vi "parking_ung2.vi"() -> ()   [LabVIEW 2012]
uses:
  G_SEN.vi
  G_NAV.vi
  G_PATH.vi
  G_VEH.vi
panel:
  out "M6006":T1={"GPSTime"=22892800.0, "attitude[2]"=-0.6123908, "lcc[0]"=-970.47205, "lcc[1]"=200.52362, "heading_GPS"=-0.6106907} {"GPSTime" format="%#_6f"}
  out "parkingpoint":dbl[][](array[numeric])=[[457.5136078182356, -783.1010211912842, 0.7436341447060439], [464.87374009628, -776.3313496446219, 0.7436341447060439], [466.7137731657911, -774.6389317579564, 0.7436341447060439], [468.5538062353022, -772.9465138712908, 0.3219638657386641], [475.6187081476555, -773.2417442369818, -0.09970641322871643], [485.5690424693232, -774.2371571598643, -0.09970641322871643]]
  out "max cost":i32=34
  out "sensor_obs":dbl[][](array[numeric])
  out "sensor_lane":dbl[][](array[numeric])=[[-17.75, -3.75, 0.0], [-17.5, -4.25, 0.0], [-17.5, -4.0, 0.0], [-17.25, -4.25, 0.0], [-14.5, -3.25, 0.0], [-14.25, -4.0, 0.0], [-14.25, -3.75, 0.0], [-14.25, -3.5, 0.0], [-13.0, -13.5, 0.0], [-12.0, -3.25, 0.0], [-11.75, -3.5, 0.0], [-11.25, 4.75, 0.0], [-11.25, 5.0, 0.0], [-10.0, -3.25, 0.0], [-9.75, -6.0, 0.0], [-9.75, -5.75, 0.0], [-9.75, -5.5, 0.0], [-9.75, 4.25, 0.0], [-9.5, -4.5, 0.0], [-9.25, -12.25, 0.0], [-9.25, -9.5, 0.0], [-9.25, -9.25, 0.0], [-9.25, -9.0, 0.0], [-9.25, -4.75, 0.0], [-9.25, -4.5, 0.0], [-9.0, -12.25, 0.0], [-9.0, -7.5, 0.0], [-9.0, -4.0, 0.0], [-8.75, -12.5, 0.0], [-8.75, -11.0, 0.0], [-8.75, 2.75, 0.0], [-8.5, -12.5, 0.0], [-8.5, -7.25, 0.0], [-8.5, -5.75, 0.0], [-8.5, -5.5, 0.0], [-8.5, -3.25, 0.0], [-8.25, 4.5, 0.0], [-7.75, 2.75, 0.0], [-7.75, 3.0, 0.0], [-7.5, -8.75, 0.0], [-7.25, -11.75, 0.0], [-7.25, -8.75, 0.0], [-7.25, 4.5, 0.0], [-7.0, -12.0, 0.0], [-7.0, -11.75, 0.0], [-7.0, -7.0, 0.0], [-7.0, -5.25, 0.0], [-6.75, -7.0, 0.0], [-6.75, -5.5, 0.0], [-6.75, 3.25, 0.0], [-6.75, 3.5, 0.0], [-6.75, 3.75, 0.0], [-6.75, 7.25, 0.0], [-6.75, 9.25, 0.0], [-6.5, -7.25, 0.0], [-6.5, 7.5, 0.0], [-6.5, 7.75, 0.0], [-6.25, -7.5, 0.0], [-6.25, -7.25, 0.0], [-6.25, 4.75, 0.0], [-6.25, 5.0, 0.0], [-6.25, 6.25, 0.0], [-6.0, -11.75, 0.0], [-6.0, -9.75, 0.0], [-6.0, -9.5, 0.0], [-6.0, 5.0, 0.0], [-5.75, -11.75, 0.0], [-5.75, -9.75, 0.0], [-5.75, -5.25, 0.0], [-5.75, -5.0, 0.0], [-5.5, -11.75, 0.0], [-5.5, -5.25, 0.0], [-5.25, -11.75, 0.0], [-5.0, -11.75, 0.0], [-5.0, -8.25, 0.0], [-5.0, -3.75, 0.0], [-4.75, -11.75, 0.0], [-4.75, -8.5, 0.0], [-4.75, -8.25, 0.0], [-4.75, -6.0, 0.0], [-4.75, -5.0, 0.0], [-4.75, -4.75, 0.0], [-4.75, -4.0, 0.0], [-4.75, -3.75, 0.0], [-4.5, -11.75, 0.0], [-4.5, -7.25, 0.0], [-4.5, -6.0, 0.0], [-4.25, -11.5, 0.0], [-4.25, -8.75, 0.0], [-4.25, -8.5, 0.0], [-4.25, -7.25, 0.0], [-4.0, -10.5, 0.0], [-4.0, -8.75, 0.0], [-3.75, -10.5, 0.0], [-2.75, -11.0, 0.0], [-2.5, -11.0, 0.0], [-2.25, -11.0, 0.0], [-2.0, -18.0, 0.0], [-2.0, -11.0, 0.0], [-1.75, -11.0, 0.0], [-1.5, -18.0, 0.0], [-1.5, -11.0, 0.0], [-1.25, -18.0, 0.0], [-1.25, -11.0, 0.0], [-1.0, -18.0, 0.0], [-1.0, -12.25, 0.0], [-1.0, -11.0, 0.0], [-0.75, -18.0, 0.0], [-0.75, -12.5, 0.0], [-0.5, -18.0, 0.0], [-0.5, -12.5, 0.0], [1.75, -12.5, 0.0], [2.0, -12.5, 0.0], [2.0, 9.0, 0.0], [2.25, 6.5, 0.0], [2.25, 7.25, 0.0], [2.5, -17.5, 0.0], [2.5, -12.25, 0.0], [2.5, 4.5, 0.0], [2.5, 5.0, 0.0], [2.5, 5.25, 0.0], [2.5, 5.5, 0.0], [2.5, 6.0, 0.0], [2.5, 6.5, 0.0], [2.5, 7.25, 0.0], [2.75, -17.5, 0.0], [2.75, -12.25, 0.0], [2.75, -10.5, 0.0], [2.75, 2.75, 0.0], [2.75, 3.0, 0.0], [2.75, 3.25, 0.0], [2.75, 3.5, 0.0], [2.75, 3.75, 0.0], [2.75, 4.0, 0.0], [2.75, 4.5, 0.0], [2.75, 4.75, 0.0], [2.75, 5.0, 0.0], [2.75, 5.25, 0.0], [2.75, 7.0, 0.0], [3.0, -12.25, 0.0], [3.0, -12.0, 0.0], [3.0, -10.5, 0.0], [3.0, 2.75, 0.0], [3.0, 3.0, 0.0], [3.0, 3.25, 0.0], [3.0, 3.5, 0.0], [3.0, 4.5, 0.0], [3.0, 4.75, 0.0], [3.25, -17.5, 0.0], [3.25, -10.5, 0.0], [3.5, -10.5, 0.0], [3.5, 4.75, 0.0], [3.75, -17.5, 0.0], [3.75, -4.75, 0.0], [3.75, -4.0, 0.0], [3.75, -3.5, 0.0], [3.75, 7.25, 0.0], [4.0, -6.25, 0.0], [4.0, -5.25, 0.0], [4.0, -4.75, 0.0], [4.0, -4.5, 0.0], [4.0, -4.0, 0.0], [4.0, 4.75, 0.0], [4.0, 5.0, 0.0], [4.0, 7.25, 0.0], [4.25, -10.25, 0.0], [4.25, -8.5, 0.0], [4.25, -5.25, 0.0], [4.5, -10.25, 0.0], [4.5, -8.5, 0.0], [4.5, 5.0, 0.0], [4.75, -17.5, 0.0], [4.75, -10.25, 0.0], [4.75, 4.75, 0.0], [4.75, 5.0, 0.0], [5.0, -17.5, 0.0], [5.0, -10.0, 0.0], [5.25, -10.0, 0.0], [5.25, 5.0, 0.0], [5.5, -10.0, 0.0], [5.5, 5.0, 0.0], [5.75, -5.0, 0.0], [6.0, -5.0, 0.0], [6.0, 5.25, 0.0], [6.25, 5.0, 0.0], [6.25, 5.25, 0.0], [6.75, -17.25, 0.0], [6.75, -17.0, 0.0], [6.75, 4.75, 0.0], [7.0, 2.75, 0.0], [7.0, 5.25, 0.0], [7.0, 5.5, 0.0], [7.25, 4.5, 0.0], [7.25, 7.75, 0.0], [7.25, 8.75, 0.0], [7.25, 9.0, 0.0], [7.5, -4.75, 0.0], [7.5, 6.0, 0.0], [7.5, 7.75, 0.0], [7.75, -4.75, 0.0], [15.0, -19.25, 0.0], [15.25, -19.25, 0.0], [15.5, -19.0, 0.0], [16.0, -19.0, 0.0], [16.0, -10.25, 0.0], [16.5, -10.25, 0.0], [16.75, -10.0, 0.0], [17.25, -10.0, 0.0], [17.5, -8.75, 0.0], [17.75, -9.75, 0.0], [17.75, -9.5, 0.0], [18.0, -9.5, 0.0], [18.0, -9.25, 0.0], [18.25, -9.25, 0.0], [18.5, -9.0, 0.0], [18.75, -9.0, 0.0], [18.75, -8.75, 0.0], [19.0, -8.75, 0.0], [19.0, -8.5, 0.0], [19.25, -8.25, 0.0], [19.5, -8.25, 0.0]]
  out "box":dbl[][](array[numeric])=[[2.75, 2.75], [7.75, 2.7499999999999996], [7.75, 5.0], [2.7500000000000004, 5.0], [2.75, 2.75]]
  out "time":u32=1
  out "tic":u32=336066801
  out "XY Graph":cluster{"Y":dbl[], "Y":dbl[]}[](graph)=[{"Y"=[2.25, 2.25, 2.5, 2.5, 2.5, 2.75, 2.75, 3.0, 3.25, 3.25, 3.5, 3.5, 4.0, 4.0, 4.5, 4.5, 4.75, 4.75, 4.75, 5.0, 5.25], "Y"=[4.25, 4.5, 4.0, 4.25, 4.5, 3.75, 4.0, 3.75, 3.5, 3.75, 3.25, 3.5, 3.0, 3.25, 2.75, 3.0, 3.25, 3.5, 4.0, 4.0, 4.5]}, {"Y"=[-25.0, -25.0, -15.0, -13.75, -10.5, -9.75, -8.5, -8.25, -8.0, -7.5, -7.25, -7.0, -7.0, -6.75, -6.5, -6.25, -6.25, -6.0, -6.0, -6.0, -5.75, -5.0, -4.75, -4.75, -4.5, -4.25, -4.25, -4.25, -4.25, -4.0, -4.0, -4.0, -4.0, -4.0, -3.75, -3.75, -3.75, -3.75, -3.5, -3.5, -3.5, -3.25, -3.25, -3.25, -3.25, -3.25, -3.0, -3.0, -3.0, -3.0, -3.0, -2.75, -2.5, -2.5, -2.5, -2.25, -2.25, -2.25, -2.0, -2.0, -2.0, -2.0, -2.0, -1.75, -1.75, -1.75, -1.75, -1.5, -1.5, -1.5, -1.5, -1.25, -1.25, -1.0, -1.0, -1.0, -0.75, -0.75, -0.75, -0.5, -0.5, -0.5, -0.25, -0.25, 0.0, 0.25, 0.25, 0.5, 0.75, 1.0, 1.0, 1.25, 1.25, 1.5, 1.5, 1.5, 1.5, 1.5, 1.5, 1.5, 1.75, 1.75, 1.75, 1.75, 1.75, 1.75, 1.75, 2.0, 2.0, 2.0, 2.0, 2.0, 2.25, 2.25, 2.25, 2.25, 2.25, 2.25, 2.25, 2.5, 2.5, 2.5, 2.5, 2.5, 2.5, 2.75, 2.75, 2.75, 2.75, 3.0, 3.0, 3.25, 3.25, 3.25, 3.25, 3.25, 3.25, 3.5, 3.5, 3.5, 3.75, 4.0, 4.0, 4.0, 4.0, 4.25, 4.25, 4.5, 4.5, 4.75, 4.75, 4.75, 5.0, 5.25, 5.25, 5.5, 5.5, 5.5, 5.5, 5.75, 5.75, 6.0, 6.0, 6.0, 6.0, 6.0, 6.25, 6.25, 6.25, 6.5, 6.5, 6.5, 6.5, 6.5, 6.5, 6.5, 6.75, 6.75, 6.75, 6.75, 6.75, 7.0, 7.0, 7.0, 7.25, 7.25, 7.25, 7.25, 7.5, 7.5, 7.5, 7.5, 7.75, 7.75, 7.75, 7.75, 8.0, 8.0, 8.0, 8.0, 8.0, 8.25, 8.25, 8.25, 8.5, 8.5, 8.5, 8.5, 8.75, 8.75, 8.75, 9.0, 9.0, 9.0, 9.0, 9.0, 9.25, 9.25, 9.25, 9.25, 9.25, 9.25, 9.5, 9.5, 9.5, 9.5, 9.5, 9.5, 9.5, 9.75, 9.75, 9.75, 9.75, 9.75, 10.0, 10.0, 10.0, 10.0, 10.0, 10.0, 10.25, 10.25, 10.25, 10.25, 10.25, 10.25, 10.5, 10.5, 10.5, 10.5, 10.75, 10.75, 10.75, 11.0, 11.0, 11.0, 11.0, 11.0, 11.25, 11.25, 11.25, 11.5, 11.75, 12.0, 14.25, 14.5, 14.75, 14.75, 14.75, 14.75, 14.75, 15.0, 15.0, 15.25, 15.25, 15.25, 15.25, 15.5, 15.5, 15.5, 15.5, 15.75, 15.75, 15.75, 16.0, 16.0, 16.25, 16.25, 16.5, 16.5, 17.0, 17.25, 17.5, 17.5, 17.75, 17.75, 17.75, 17.75, 18.0, 18.0, 18.0, 18.0, 18.0, 18.0, 18.0, 18.0, 18.25, 18.25, 18.25, 18.25, 18.5, 18.5, 18.5, 18.75, 18.75, 18.75, 19.0, 19.0, 19.0, 19.0, 19.0, 19.25, 19.25, 19.25, 19.25, 19.25, 19.25, 19.25, 19.5, 19.5, 19.5, 19.5, 19.5, 19.5, 19.5, 19.75, 19.75, 19.75, 19.75, 19.75, 19.75, 20.0, 20.0, 20.0, 20.0, 20.0, 20.0, 20.25, 20.25, 20.25, 20.25, 20.25, 20.5, 20.5, 20.5, 20.75, 20.75, 21.0, 21.0, 21.0, 21.5, 21.5, 21.5, 21.5, 22.0, 22.25, 22.5, 22.5, 22.5, 22.5, 22.75, 22.75, 23.0, 23.25, 23.5, 23.75, 24.0, 24.0, 24.0, 24.0, 24.25, 24.25, 24.5, 24.5, 24.75, 24.75, 24.75, -1.75, -1.25, -1.0, -0.5, 0.0, -3.0, -3.0, -1.75, 0.25], "Y"=[6.5, 22.75, -12.0, -8.5, -4.25, -13.75, -11.0, -11.25, -11.25, 9.5, -9.25, -9.5, -9.25, -9.5, -7.75, -8.0, 8.75, -8.0, -6.75, 8.75, -6.75, 8.0, -6.25, 8.0, -5.25, -5.5, -5.25, 13.5, 13.75, -4.75, 7.5, 8.5, 8.75, 13.5, -4.25, 7.5, 8.75, 13.25, -3.75, 13.0, 13.25, -7.5, -3.5, -3.25, 7.0, 13.0, -8.5, -8.0, -7.5, 7.0, 7.25, -8.0, -7.75, -7.0, 6.75, -6.25, -3.25, 6.75, -6.25, -5.5, -3.25, 6.75, 7.0, -5.5, -5.0, -3.5, 6.25, -5.0, -4.75, -3.5, 7.75, -4.75, -4.25, -9.25, -7.25, -4.25, -7.25, -6.25, 5.75, -9.25, -7.25, -6.25, -9.25, 5.5, 5.5, 5.25, 5.5, 5.0, -5.0, -7.0, -5.0, -10.75, -6.25, -13.5, -13.25, -11.25, -10.25, -6.25, -6.0, -5.5, -13.0, -11.5, -11.25, -10.75, -9.0, -7.75, -5.5, -12.75, -11.5, -10.75, -9.0, -7.75, -11.5, -11.25, -10.5, -6.0, -5.75, 4.25, 4.5, -11.25, -10.5, -5.75, 4.0, 4.25, 4.5, -11.0, -10.25, 3.75, 4.0, -6.5, 3.75, -9.5, -6.5, -6.25, 3.5, 3.75, 6.0, -9.0, 3.25, 3.5, 7.0, -7.0, 3.0, 3.25, 7.75, -7.0, 7.75, 2.75, 3.0, 3.25, 3.5, 4.0, 4.0, -5.0, 4.5, -5.0, -4.75, 5.0, 5.25, -4.75, -4.5, -5.0, -4.5, -4.25, 6.0, 6.75, -5.0, -4.25, -4.0, -19.25, -19.0, -4.0, -3.75, -3.5, 6.75, 7.0, -19.0, -18.75, -3.5, -3.25, 7.5, -19.0, -5.25, 7.25, -19.0, -18.75, -5.25, -5.0, -18.75, -18.25, -5.0, -4.75, -18.25, -18.0, -4.75, -4.5, -18.0, -17.75, -5.75, -4.25, -4.0, -5.5, -4.0, -3.75, -5.25, -5.0, -3.5, -3.25, -17.25, -6.75, -4.75, -13.25, -6.75, -6.5, -4.75, -4.5, -13.0, -12.75, -6.5, -6.25, -4.25, -4.0, -12.75, -12.5, -8.75, -6.0, -4.0, -3.75, -3.5, -12.5, -12.25, -5.75, -5.5, -3.25, -12.25, -12.0, -5.5, -5.25, 2.75, 3.0, -12.0, -11.75, -11.5, -5.25, -5.0, -4.75, -11.5, -11.25, -4.75, -4.5, -11.0, -4.5, -4.25, -10.75, -10.5, -10.25, -3.75, -3.5, -10.25, -10.0, -3.25, -10.0, -6.0, -6.0, -13.25, -13.0, -13.0, -12.75, -12.5, -5.75, -5.5, -12.5, -5.5, -12.25, -12.0, -4.75, -4.5, -12.0, -11.75, -4.5, -4.25, -11.25, -4.25, -4.0, -10.75, -3.75, -10.5, -10.25, -10.25, -10.0, -9.5, 16.75, -8.75, 16.75, -8.75, 16.25, 16.5, 16.75, -8.5, -8.25, -8.0, 15.25, 15.5, 15.75, 16.0, 16.25, -8.0, -7.75, 15.25, 15.5, 2.75, 15.0, 15.25, -7.5, 3.0, 15.0, -7.25, -7.0, 3.5, 3.75, 4.0, -19.25, -6.75, -6.5, -6.25, 4.0, 4.25, 4.5, -19.25, -19.0, -18.75, -18.25, -6.5, -6.25, 4.5, -18.5, -18.25, -18.0, -17.75, 4.75, 5.0, -17.75, -17.25, -5.0, 5.25, 5.5, 5.75, -16.75, -5.0, 5.75, 6.0, 6.25, -16.75, -4.75, 6.5, -16.5, -4.5, -16.0, -15.75, -4.25, -15.25, -15.0, -4.0, -3.75, -15.0, -14.75, -14.75, -14.5, -14.25, -14.0, -14.0, -13.75, -13.5, -13.5, -12.25, -12.0, -12.0, -11.75, -11.5, -11.25, -11.75, -11.25, -11.0, 5.0, -10.0, 22.75, 23.0, 6.5, 6.0, 6.0, 5.75, 5.75, 10.25, 10.5, 7.75, 5.75]}, {"Y"=[1.0, 1.0, 1.0, 1.0, 1.0, 1.0, 1.0, 1.0, 1.0, 1.0, 1.0, 1.0, 1.0, 1.0, 1.0, 1.25, 1.25, 1.25, 1.25, 1.25, 1.25, 1.25, 1.25, 1.25, 1.25, 1.25, 1.25, 1.25, 1.25, 1.25, 1.25, 1.5, 1.5, 1.5, 1.5, 1.5, 1.5, 1.5, 1.5, 1.5, 1.5, 1.5, 1.5, 1.75, 1.75, 1.75, 1.75, 1.75, 1.75, 1.75, 1.75, 2.0, 2.0, 2.0, 2.0, 2.0, 2.0, 2.0, 2.0, 2.25, 2.25, 2.25, 2.25, 2.25, 2.25, 2.25, 2.25, 2.5, 2.5, 2.5, 2.5, 2.5, 2.5, 2.5, 2.5, 2.5, 2.5, 2.75, 2.75, 2.75, 2.75, 2.75, 2.75, 2.75, 2.75, 2.75, 2.75, 3.0, 3.0, 3.0, 3.0, 3.0, 3.0, 3.25, 3.25, 3.25, 3.5, 3.5, 3.5, 3.5, 3.75], "Y"=[5.0, 5.25, 5.5, 5.75, 6.0, 6.5, 7.0, 7.5, 7.75, 8.0, 8.25, 8.5, 9.0, 9.25, 9.5, 4.75, 5.0, 5.25, 5.5, 5.75, 6.0, 6.25, 6.5, 6.75, 7.5, 7.75, 8.0, 8.25, 8.5, 8.75, 9.0, 4.75, 5.0, 5.25, 5.5, 5.75, 6.0, 6.25, 6.5, 6.75, 8.5, 8.75, 9.0, 4.75, 5.0, 5.25, 5.5, 5.75, 6.75, 7.5, 9.0, 4.75, 5.0, 5.25, 5.5, 5.75, 6.75, 7.0, 7.5, 4.75, 5.0, 5.25, 5.5, 5.75, 6.5, 6.75, 7.5, 4.75, 5.0, 5.25, 5.5, 5.75, 6.0, 6.5, 7.25, 7.5, 9.75, 4.75, 5.0, 5.25, 5.5, 5.75, 6.0, 6.25, 6.5, 7.0, 7.25, 5.5, 6.0, 6.5, 6.75, 7.0, 7.25, 6.5, 6.75, 7.0, 6.5, 7.25, 7.5, 7.75, 7.25]}, {"Y"=[-24.75, -24.75, -24.75, -24.75, -24.5, -24.5, -24.5, -24.5, -24.25, -24.25, -24.25, -24.25, -24.25, -24.0, -24.0, -24.0, -24.0, -24.0, -24.0, -24.0, -24.0, -24.0, -23.75, -23.75, -23.75, -23.75, -23.75, -23.75, -23.75, -23.5, -23.5, -23.5, -23.5, -23.5, -23.5, -23.5, -23.5, -23.5, -23.5, -23.5, -23.25, -23.25, -23.25, -23.25, -23.25, -23.25, -23.25, -23.25, -23.25, -23.25, -23.0, -23.0, -23.0, -23.0, -23.0, -23.0, -23.0, -23.0, -22.75, -22.75, -22.75, -22.75, -22.75, -22.75, -22.75, -22.75, -22.75, -22.75, -22.5, -22.5, -22.5, -22.5, -22.5, -22.5, -22.5, -22.5, -22.5, -22.5, -22.5, -22.5, -22.5, -22.5, -22.25, -22.25, -22.25, -22.25, -22.25, -22.25, -22.25, -22.25, -22.25, -22.25, -22.25, -22.25, -22.25, -22.25, -22.25, -22.25, -22.25, -22.0, -22.0, -22.0, -22.0, -22.0, -22.0, -22.0, -22.0, -22.0, -22.0, -22.0, -21.75, -21.75, -21.75, -21.75, -21.5, -21.5, -21.5, -21.25, -21.25, -21.25, -21.25, -21.25, -21.0, -21.0, -21.0, -21.0, -21.0, -20.75, -20.75, -20.75, -20.75, -20.75, -20.75, -20.75, -20.5, -20.5, -20.0, -20.0, -19.75, -19.5, -19.25, -19.25, -19.25, -19.25, -19.0, -19.0, -19.0, -19.0, -18.75, -18.75, -18.75, -18.75, -18.75, -18.75, -18.5, -18.5, -18.5, -18.5, -18.5, -18.5, -18.5, -18.5, -18.5, -18.5, -18.5, -18.25, -18.25, -18.25, -18.25, -18.25, -18.25, -18.25, -18.25, -18.25, -18.25, -18.25, -18.25, -18.25, -18.25, -18.25, -18.0, -18.0, -18.0, -18.0, -18.0, -18.0, -18.0, -18.0, -18.0, -18.0, -18.0, -18.0, -18.0, -18.0, -18.0, -17.75, -17.75, -17.75, -17.75, -17.75, -17.75, -17.75, -17.75, -17.75, -17.75, -17.5, -17.5, -17.5, -17.5, -17.5, -17.5, -17.5, -17.5, -17.5, -17.5, -17.5, -17.25, -17.25, -17.25, -17.25, -17.25, -17.25, -17.25, -17.25, -17.25, -17.0, -17.0, -17.0, -17.0, -16.75, -16.75, -16.5, -16.0, -16.0, -16.0, -16.0, -15.75, -15.75, -15.75, -15.75, -15.75, -15.75, -15.75, -15.75, -15.75, -15.5, -15.5, -15.5, -15.5, -15.5, -15.5, -15.5, -15.5, -15.5, -15.25, -15.25, -15.25, -15.25, -15.25, -15.25, -15.25, -15.25, -15.0, -15.0, -15.0, -15.0, -15.0, -15.0, -15.0, -15.0, -15.0, -15.0, -14.75, -14.75, -14.75, -14.75, -14.75, -14.75, -14.75, -14.75, -14.75, -14.5, -14.5, -14.5, -14.25, -14.25, -14.25, -14.25, -14.0, -14.0, -14.0, -14.0, -14.0, -13.75, -13.75, -13.75, -13.75, -13.75, -13.75, -13.75, -13.75, -13.75, -13.5, -13.5, -13.5, -13.5, -13.5, -13.5, -13.5, -13.25, -13.25, -13.25, -13.25, -13.25, -13.25, -13.25, -13.0, -13.0, -13.0, -13.0, -13.0, -12.75, -12.75, -12.75, -12.75, -12.5, -12.5, -12.5, -12.5, -12.5, -12.5, -12.5, -12.5, -12.5, -12.25, -12.25, -12.25, -12.25, -12.25, -12.25, -12.25, -12.25, -12.25, -12.25, -12.25, -12.25, -12.25, -12.25, -12.25, -12.25, -12.25, -12.0, -12.0, -12.0, -12.0, -12.0, -12.0, -12.0, -12.0, -12.0, -12.0, -12.0, -12.0, -11.75, -11.75, -11.75, -11.75, -11.75, -11.75, -11.75, -11.75, -11.75, -11.75, -11.75, -11.75, -11.75, -11.75, -11.75, -11.75, -11.75, -11.75, -11.5, -11.5, -11.5, -11.5, -11.5, -11.5, -11.5, -11.5, -11.5, -11.5, -11.5, -11.25, -11.25, -11.25, -11.25, -11.25, -11.25, -11.25, -11.25, -11.25, -11.0, -11.0, -11.0, -11.0, -11.0, -11.0, -11.0, -11.0, -11.0, -11.0, -11.0, -11.0, -10.75, -10.75, -10.75, -10.75, -10.75, -10.75, -10.75, -10.75, -10.75, -10.75, -10.75, -10.5, -10.5, -10.5, -10.5, -10.5, -10.5, -10.5, -10.25, -10.25, -10.25, -10.25, -10.25, -10.0, -10.0, -10.0, -10.0, -10.0, -9.75, -9.75, -9.75, -9.5, -9.5, -9.25, -9.25, -9.25, -9.0, -9.0, -9.0, -9.0, -8.75, -8.75, -8.75, -8.75, -8.5, -8.5, -8.5, -8.25, -8.25, -8.25, -8.25, -8.25, -8.25, -8.0, -8.0, -8.0, -8.0, -8.0, -8.0, -7.75, -7.75, -7.75, -7.75, -7.75, -7.5, -7.5, -7.5, -7.5, -7.5, -7.5, -7.25, -7.25, -7.25, -7.25, -7.25, -7.0, -7.0, -7.0, -7.0, -7.0, -7.0, -7.0, -7.0, -7.0, -6.75, -6.75, -6.75, -6.75, -6.75, -6.5, -6.5, -6.5, -6.5, -6.5, -6.25, -6.25, -6.25, -6.25, -6.25, -6.0, -6.0, -6.0, -6.0, -6.0, -6.0, -5.75, -5.75, -5.75, -5.75, -5.75, -5.75, -5.75, -5.75, -5.75, -5.75, -5.75, -5.5, -5.5, -5.5, -5.5, -5.5, -5.5, -5.5, -5.5, -5.5, -5.5, -5.5, -5.5, -5.5, -5.5, -5.25, -5.25, -5.25, -5.25, -5.25, -5.25, -5.25, -5.25, -5.25, -5.25, -5.25, -5.0, -5.0, -5.0, -5.0, -5.0, -5.0, -5.0, -5.0, -5.0, -5.0, -5.0, -4.75, -4.75, -4.75, -4.75, -4.75, -4.75, -4.75, -4.75, -4.75, -4.75, -4.75, -4.75, -4.75, -4.75, -4.75, -4.5, -4.5, -4.5, -4.5, -4.5, -4.5, -4.5, -4.5, -4.5, -4.25, -4.25, -4.25, -4.25, -4.25, -4.25, -4.25, -4.25, -4.0, -4.0, -4.0, -4.0, -4.0, -4.0, -4.0, -4.0, -4.0, -4.0, -4.0, -3.75, -3.75, -3.75, -3.75, -3.75, -3.75, -3.75, -3.75, -3.75, -3.75, -3.75, -3.5, -3.5, -3.5, -3.5, -3.5, -3.5, -3.5, -3.5, -3.5, -3.25, -3.25, -3.25, -3.25, -3.25, -3.25, -3.25, -3.25, -3.25, -3.25, -3.25, -3.25, -3.0, -3.0, -3.0, -3.0, -3.0, -3.0, -3.0, -3.0, -3.0, -3.0, -3.0, -2.75, -2.75, -2.75, -2.75, -2.75, -2.75, -2.75, -2.75, -2.75, -2.75, -2.75, -2.75, -2.75, -2.75, -2.75, -2.5, -2.5, -2.5, -2.5, -2.5, -2.5, -2.5, -2.5, -2.5, -2.5, -2.5, -2.5, -2.25, -2.25, -2.25, -2.25, -2.25, -2.25, -2.25, -2.25, -2.25, -2.25, -2.25, -2.25, -2.0, -2.0, -2.0, -2.0, -2.0, -2.0, -2.0, -2.0, -2.0, -2.0, -2.0, -2.0, -2.0, -2.0, -2.0, -1.75, -1.75, -1.75, -1.75, -1.75, -1.75, -1.75, -1.75, -1.75, -1.75, -1.75, -1.75, -1.5, -1.5, -1.5, -1.5, -1.5, -1.5, -1.5, -1.5, -1.5, -1.5, -1.5, -1.5, -1.5, -1.5, -1.5, -1.5, -1.5, -1.5, -1.25, -1.25, -1.25, -1.25, -1.25, -1.25, -1.25, -1.25, -1.25, -1.25, -1.25, -1.25, -1.25, -1.25, -1.25, -1.25, -1.0, -1.0, -1.0, -1.0, -1.0, -1.0, -1.0, -1.0, -1.0, -1.0, -1.0, -1.0, -1.0, -1.0, -0.75, -0.75, -0.75, -0.75, -0.75, -0.75, -0.75, -0.75, -0.75, -0.75, -0.75, -0.75, -0.75, -0.75, -0.5, -0.5, -0.5, -0.5, -0.5, -0.5, -0.5, -0.5, -0.5, -0.5, -0.5, -0.5, -0.5, -0.5, -0.25, -0.25, -0.25, -0.25, -0.25, -0.25, -0.25, -0.25, -0.25, -0.25, 0.0, 0.0, 0.0, 0.0, 0.0, 0.0, 0.0, 0.0, 0.0, 0.0, 0.0, 0.0, 0.25, 0.25, 0.25, 0.25, 0.25, 0.25, 0.25, 0.25, 0.25, 0.25, 0.25, 0.25, 0.25, 0.5, 0.5, 0.5, 0.5, 0.5, 0.5, 0.5, 0.5, 0.5, 0.5, 0.75, 0.75, 0.75, 0.75, 0.75, 0.75, 0.75, 0.75, 0.75, 0.75, 0.75, 0.75, 0.75, 1.0, 1.0, 1.0, 1.0, 1.0, 1.0, 1.0, 1.0, 1.0, 1.0, 1.0, 1.0, 1.0, 1.0, 1.0, 1.25, 1.25, 1.25, 1.25, 1.25, 1.25, 1.25, 1.25, 1.25, 1.25, 1.25, 1.25, 1.25, 1.25, 1.25, 1.25, 1.25, 1.25, 1.5, 1.5, 1.5, 1.5, 1.5, 1.5, 1.5, 1.5, 1.5, 1.5, 1.5, 1.5, 1.5, 1.5, 1.75, 1.75, 1.75, 1.75, 1.75, 1.75, 1.75, 1.75, 1.75, 1.75, 1.75, 1.75, 1.75, 2.0, 2.0, 2.0, 2.0, 2.0, 2.0, 2.0, 2.0, 2.0, 2.0, 2.0, 2.0, 2.0, 2.0, 2.0, 2.0, 2.0, 2.0, 2.25, 2.25, 2.25, 2.25, 2.25, 2.25, 2.25, 2.25, 2.25, 2.25, 2.25, 2.25, 2.25, 2.25, 2.25, 2.25, 2.25, 2.25, 2.5, 2.5, 2.5, 2.5, 2.5, 2.5, 2.5, 2.5, 2.5, 2.5, 2.5, 2.5, 2.5, 2.5, 2.5, 2.5, 2.5, 2.5, 2.5, 2.75, 2.75, 2.75, 2.75, 2.75, 2.75, 2.75, 2.75, 2.75, 2.75, 2.75, 2.75, 2.75, 2.75, 2.75, 2.75, 2.75, 2.75, 2.75, 2.75, 2.75, 3.0, 3.0, 3.0, 3.0, 3.0, 3.0, 3.0, 3.0, 3.0, 3.0, 3.0, 3.0, 3.0, 3.0, 3.0, 3.25, 3.25, 3.25, 3.25, 3.25, 3.25, 3.25, 3.25, 3.25, 3.25, 3.25, 3.25, 3.25, 3.5, 3.5, 3.5, 3.5, 3.5, 3.5, 3.5, 3.5, 3.5, 3.5, 3.5, 3.5, 3.5, 3.5, 3.5, 3.75, 3.75, 3.75, 3.75, 3.75, 3.75, 3.75, 3.75, 3.75, 3.75, 3.75, 4.0, 4.0, 4.0, 4.0, 4.0, 4.0, 4.0, 4.0, 4.0, 4.0, 4.25, 4.25, 4.25, 4.25, 4.25, 4.25, 4.25, 4.25, 4.25, 4.5, 4.5, 4.5, 4.5, 4.5, 4.5, 4.5, 4.5, 4.5, 4.5, 4.5, 4.75, 4.75, 4.75, 4.75, 4.75, 4.75, 4.75, 4.75, 4.75, 4.75, 5.0, 5.0, 5.0, 5.0, 5.0, 5.0, 5.0, 5.0, 5.0, 5.0, 5.0, 5.0, 5.25, 5.25, 5.25, 5.25, 5.25, 5.25, 5.25, 5.25, 5.25, 5.25, 5.25, 5.25, 5.25, 5.25, 5.25, 5.5, 5.5, 5.5, 5.5, 5.5, 5.5, 5.5, 5.5, 5.5, 5.5, 5.5, 5.5, 5.5, 5.5, 5.5, 5.5, 5.5, 5.5, 5.5, 5.5, 5.5, 5.5, 5.5, 5.75, 5.75, 5.75, 5.75, 5.75, 5.75, 5.75, 5.75, 5.75, 5.75, 5.75, 5.75, 5.75, 5.75, 5.75, 5.75, 5.75, 5.75, 5.75, 5.75, 5.75, 5.75, 5.75, 5.75, 5.75, 5.75, 6.0, 6.0, 6.0, 6.0, 6.0, 6.0, 6.0, 6.0, 6.0, 6.0, 6.0, 6.0, 6.0, 6.0, 6.0, 6.0, 6.0, 6.0, 6.0, 6.0, 6.0, 6.0, 6.0, 6.0, 6.0, 6.25, 6.25, 6.25, 6.25, 6.25, 6.25, 6.25, 6.25, 6.25, 6.25, 6.25, 6.25, 6.25, 6.25, 6.5, 6.5, 6.5, 6.5, 6.5, 6.5, 6.5, 6.5, 6.5, 6.5, 6.5, 6.5, 6.5, 6.5, 6.5, 6.5, 6.5, 6.5, 6.5, 6.5, 6.5, 6.5, 6.75, 6.75, 6.75, 6.75, 6.75, 6.75, 6.75, 6.75, 6.75, 6.75, 6.75, 6.75, 6.75, 6.75, 6.75, 6.75, 6.75, 7.0, 7.0, 7.0, 7.0, 7.0, 7.0, 7.0, 7.0, 7.0, 7.0, 7.0, 7.0, 7.0, 7.0, 7.0, 7.0, 7.0, 7.25, 7.25, 7.25, 7.25, 7.25, 7.25, 7.25, 7.25, 7.25, 7.25, 7.25, 7.25, 7.25, 7.25, 7.25, 7.5, 7.5, 7.5, 7.5, 7.5, 7.5, 7.5, 7.5, 7.5, 7.5, 7.5, 7.5, 7.5, 7.75, 7.75, 7.75, 7.75, 7.75, 7.75, 7.75, 7.75, 7.75, 7.75, 7.75, 7.75, 7.75, 7.75, 8.0, 8.0, 8.0, 8.0, 8.0, 8.0, 8.0, 8.0, 8.25, 8.25, 8.25, 8.25, 8.25, 8.25, 8.25, 8.5, 8.5, 8.5, 8.5, 8.5, 8.5, 8.5, 8.5, 8.5, 8.75, 8.75, 8.75, 8.75, 8.75, 8.75, 8.75, 8.75, 8.75, 8.75, 8.75, 8.75, 9.0, 9.0, 9.0, 9.0, 9.0, 9.0, 9.0, 9.0, 9.0, 9.0, 9.0, 9.0, 9.0, 9.0, 9.0, 9.25, 9.25, 9.25, 9.25, 9.25, 9.25, 9.25, 9.25, 9.25, 9.25, 9.25, 9.25, 9.25, 9.25, 9.25, 9.25, 9.25, 9.25, 9.25, 9.25, 9.25, 9.5, 9.5, 9.5, 9.5, 9.5, 9.5, 9.5, 9.5, 9.5, 9.5, 9.5, 9.5, 9.5, 9.5, 9.75, 9.75, 9.75, 9.75, 9.75, 10.0, 10.0, 10.0, 10.0, 10.0, 10.25, 10.25, 10.25, 10.25, 10.25, 10.25, 10.25, 10.25, 10.25, 10.25, 10.25, 10.25, 10.5, 10.5, 10.5, 10.5, 10.5, 10.5, 10.5, 10.5, 10.5, 10.5, 10.5, 10.5, 10.75, 10.75, 10.75, 10.75, 10.75, 10.75, 10.75, 10.75, 10.75, 11.0, 11.0, 11.0, 11.0, 11.0, 11.0, 11.0, 11.25, 11.25, 11.25, 11.25, 11.25, 11.25, 11.25, 11.25, 11.25, 11.5, 11.5, 11.5, 11.5, 11.5, 11.75, 11.75, 11.75, 11.75, 12.0, 12.0, 12.0, 12.0, 12.0, 12.0, 12.0, 12.0, 12.0, 12.25, 12.25, 12.25, 12.25, 12.25, 12.25, 12.25, 12.25, 12.25, 12.25, 12.25, 12.25, 12.25, 12.25, 12.5, 12.5, 12.5, 12.5, 12.5, 12.5, 12.5, 12.5, 12.5, 12.5, 12.5, 12.75, 12.75, 13.0, 13.0, 13.25, 15.0, 15.25, 15.25, 15.25, 15.5, 15.5, 15.5, 15.75, 16.75, 16.75, 17.0, 17.0, 18.0, 18.0, 18.0, 18.25, 18.25, 18.25, 18.5, 20.75, 20.75, 21.0, 22.75, 22.75, 23.0, 23.0, 23.0, 23.25, 23.25, 23.25, 23.25, 23.5, 23.5, 23.5, 23.5, 23.5, 23.5, 23.5, 23.5, 23.5, 23.5, 23.5, 23.75, 23.75, 23.75, 23.75, 23.75, 23.75, 23.75, 23.75, 23.75, 23.75, 23.75, 23.75, 24.0, 24.0, 24.0, 24.0, 24.0, 24.0, 24.25, 24.25, 24.25, 24.5, 24.5, 24.5], "Y"=[10.25, 10.5, 10.75, 11.0, 10.75, 11.0, 11.25, 11.5, 11.0, 11.25, 11.5, 11.75, 35.5, 10.5, 10.75, 11.0, 11.25, 11.75, 12.0, 12.25, 35.25, 35.5, 10.5, 10.75, 11.0, 12.25, 12.5, 12.75, 35.25, -26.0, 10.5, 10.75, 11.0, 11.25, 11.5, 12.5, 12.75, 13.0, 35.25, 35.5, -26.0, -25.75, 5.75, 6.0, 6.25, 11.25, 13.0, 13.25, 13.5, 35.25, -26.0, 6.0, 6.25, 6.5, 6.75, 13.5, 13.75, 14.0, 6.5, 6.75, 7.0, 13.75, 14.0, 14.25, 14.5, 18.5, 18.75, 19.0, 7.0, 7.25, 7.5, 8.75, 9.0, 14.5, 14.75, 18.5, 18.75, 19.0, 19.25, 19.5, 35.25, 35.5, -6.5, -6.25, -6.0, 7.5, 7.75, 8.0, 8.5, 8.75, 14.25, 14.75, 15.0, 15.25, 19.25, 19.75, 35.5, 35.75, 36.0, -6.25, 8.0, 8.25, 8.5, 8.75, 15.25, 15.5, 15.75, 35.75, 36.0, 36.5, -6.5, -6.25, 15.75, 36.25, -6.75, -6.5, 15.0, -6.75, 15.0, 15.25, 36.5, 38.75, 15.0, 15.25, 36.25, 39.0, 39.25, 15.0, 15.25, 15.5, 15.75, 16.0, 16.25, 36.5, 15.25, 15.5, 36.75, 37.0, 36.75, 20.25, -13.5, 20.0, 20.25, 20.5, -13.75, -13.5, 20.25, 20.75, -16.25, -13.5, 20.25, 20.5, 20.75, 21.0, -17.25, -16.5, -16.25, -14.0, -13.75, 15.5, 20.25, 20.5, 20.75, 21.0, 21.5, -17.5, -17.25, -16.5, -16.25, -14.0, -13.75, 15.5, 15.75, 20.25, 20.5, 20.75, 21.0, 21.25, 21.5, 21.75, -17.25, -17.0, -16.75, -16.5, -14.25, -14.0, 4.0, 4.25, 4.5, 4.75, 15.75, 16.0, 20.5, 20.75, 21.25, -17.25, -17.0, -15.25, -15.0, -14.25, 4.0, 4.5, 16.25, 16.5, 16.75, -15.0, -14.75, -14.5, -14.25, 3.5, 3.75, 4.25, 4.5, 16.5, 16.75, 17.0, -14.5, 3.75, 4.0, 4.25, 17.0, 17.25, 17.5, 17.75, 37.25, 4.0, 4.25, 17.75, 37.5, -4.0, 37.5, -4.0, 0.75, 1.0, 1.75, 2.0, 1.0, 1.25, 1.75, 2.75, 3.0, 3.25, 3.5, 3.75, 4.0, -11.25, 1.5, 1.75, 2.0, 2.25, 2.75, 3.25, 3.75, 37.75, -11.25, 2.0, 2.25, 2.5, 2.75, 3.5, 3.75, 37.75, -10.75, -10.25, -10.0, 2.5, 2.75, 3.0, 3.25, 3.5, 37.5, 37.75, -10.75, -10.5, -10.25, -10.0, -3.75, -3.5, -3.25, 3.0, 3.25, -10.25, -3.75, -3.5, -4.0, -3.75, 41.25, 41.5, -8.25, -7.5, -4.25, -4.0, 41.25, -9.0, -8.0, -7.75, -7.5, -4.5, -4.25, -4.0, 41.25, 41.5, -9.0, -8.75, -8.0, -7.75, -4.75, -4.5, -4.25, -8.75, -8.5, -8.25, -8.0, -4.75, -4.5, -4.25, -17.0, -9.0, -8.75, -5.0, -4.5, -17.0, -16.75, -4.75, -4.5, -17.0, -16.75, -6.25, -5.75, -5.5, -5.0, -4.75, -1.25, -1.0, -17.0, -16.75, -6.5, -6.25, -6.0, -5.75, -5.25, -5.0, -4.75, -2.75, -2.5, -2.25, -2.0, -1.75, -1.5, -1.25, -1.0, -17.75, -17.25, -17.0, -6.5, -6.25, -6.0, -5.5, -5.25, -5.0, -2.5, -2.25, -2.0, -18.0, -17.75, -17.5, -17.25, -17.0, -6.5, -6.25, -6.0, -5.75, -5.5, -5.25, -5.0, -2.75, -2.5, -2.0, -1.75, -1.5, -1.25, -18.25, -18.0, -17.75, -17.5, -17.25, -5.5, -1.5, -1.25, -1.0, -0.5, 1.25, -1.25, -1.0, -0.75, -0.5, -0.25, 0.0, 1.0, 1.25, 29.75, -18.75, -18.5, -0.75, -0.5, -0.25, 0.5, 0.75, 1.0, 1.25, 1.5, 29.5, 29.75, -18.75, -18.5, -0.5, -0.25, 0.0, 0.25, 0.5, 0.75, 1.0, 29.5, 30.0, -19.0, -18.75, 0.0, 0.25, 0.5, 0.75, 29.5, -19.25, -19.0, 29.25, 29.5, 29.75, -19.25, -19.0, 29.25, 29.5, 29.75, -19.5, -19.25, 29.75, -19.5, -19.25, -19.75, -19.5, 21.5, -19.75, 21.25, 21.5, 21.75, 17.25, 17.5, 21.25, 21.5, 17.5, 17.75, 40.0, 17.25, 17.5, 17.75, 18.25, 18.5, 40.25, 17.25, 17.5, 17.75, 18.25, 18.5, 18.75, 10.0, 17.25, 18.25, 18.5, 18.75, 9.75, 10.0, 10.25, 17.5, 17.75, 18.25, 9.75, 10.0, 10.25, 17.5, 17.75, 9.75, 10.0, 10.25, 17.5, 17.75, 18.0, 24.0, 24.25, 40.5, 9.75, 10.0, 10.25, 24.0, 40.75, 10.0, 10.25, 10.5, 40.75, 41.0, 10.25, 10.5, 10.75, 11.0, 11.75, 10.75, 11.0, 11.25, 11.5, 11.75, 12.25, -7.0, 10.75, 11.0, 11.25, 11.5, 11.75, 12.0, 12.25, 20.5, 20.75, 21.25, -7.25, -7.0, 11.0, 11.5, 11.75, 12.0, 12.25, 12.5, 12.75, 20.0, 20.5, 20.75, 21.0, 21.25, -17.0, -7.5, -7.25, -7.0, 11.25, 12.0, 12.25, 12.5, 12.75, 20.25, 21.25, -17.0, -16.75, -7.5, 12.5, 12.75, 13.0, 13.25, 13.75, 16.0, 21.0, 21.25, -17.0, -16.75, -16.5, -7.75, -7.5, 12.75, 13.0, 13.25, 13.5, 13.75, 15.75, 16.0, 16.25, 21.0, 21.25, -17.0, -16.75, -16.25, -7.75, 13.75, 16.25, 16.5, 21.0, 21.25, -16.5, -16.0, -15.75, -8.0, -7.75, 14.5, 16.25, 41.5, -16.0, -8.0, -7.75, 14.25, 14.5, 14.75, 15.25, 16.25, 16.5, 41.75, 42.0, -15.0, -14.75, -8.0, -7.75, 14.25, 14.5, 14.75, 15.0, 16.25, 41.5, 41.75, -15.25, -15.0, -14.75, -14.25, 14.25, 14.5, 14.75, 41.5, 41.75, -14.5, -14.0, -13.75, -13.5, -13.25, -6.75, 14.0, 14.25, 14.5, 15.0, 15.5, 41.75, -14.0, -13.75, -13.5, -13.25, -7.0, -6.75, 14.0, 14.5, 14.75, 15.25, 15.5, -14.0, -13.75, -13.5, -13.25, -13.0, -8.75, -8.5, -7.0, 13.75, 14.0, 14.25, 14.5, 15.5, 15.75, 41.0, -13.5, -12.75, -12.5, -12.25, -8.75, 13.75, 14.0, 14.25, 14.5, 15.75, 40.75, 41.0, -13.0, -12.25, -12.0, -9.5, -9.0, -8.75, 13.75, 14.0, 14.25, 14.5, 40.75, 41.0, -12.5, -12.25, -12.0, -11.75, -11.5, -11.25, -11.0, -9.5, -9.25, -9.0, 13.75, 14.0, 14.25, 41.0, 41.25, -12.25, -12.0, -11.75, -11.5, -11.25, -11.0, -9.5, -9.25, 14.0, 14.25, 41.0, 41.5, -12.0, -11.75, -11.5, -11.25, -11.0, -10.75, -9.5, -9.25, 6.5, 7.0, 12.25, 12.5, 14.25, 14.5, 15.0, 15.25, 41.25, 44.25, -11.75, -11.5, -11.25, -11.0, -10.75, -9.25, 6.5, 6.75, 7.0, 12.25, 12.5, 15.0, 15.25, 43.0, 44.25, 44.5, -12.0, -11.75, -11.5, -11.25, -11.0, 6.5, 6.75, 7.0, 15.0, 15.25, 15.5, 42.75, 44.5, 44.75, -12.0, -11.75, -11.5, -11.25, -11.0, 6.0, 6.5, 6.75, 7.0, 7.25, 7.5, 7.75, 44.5, 44.75, -12.0, -11.75, -11.5, -11.25, 6.0, 6.25, 6.5, 6.75, 7.0, 7.25, 7.75, 44.5, 44.75, 45.0, -12.0, -11.5, -11.25, 6.0, 6.25, 6.5, 7.0, 8.0, 8.5, 44.75, -11.5, -11.25, -10.25, -10.0, 6.0, 6.25, 6.5, 7.0, 8.5, 20.75, 21.0, 21.25, -21.5, -21.25, -11.25, -10.25, 6.0, 6.25, 6.5, 6.75, 7.0, 20.75, 21.0, 21.25, 24.5, -10.75, 6.0, 6.5, 6.75, 7.0, 7.25, 7.75, 20.75, 21.0, 24.75, -10.75, 5.0, 5.25, 5.75, 6.0, 6.5, 7.0, 7.25, 7.5, 7.75, 8.0, 20.75, 21.0, 5.0, 5.25, 5.5, 5.75, 6.0, 6.5, 7.0, 7.5, 7.75, 8.0, 8.25, 8.5, 9.0, 9.25, 9.5, -16.75, 4.75, 5.0, 5.25, 5.5, 5.75, 6.0, 6.25, 6.5, 6.75, 7.5, 7.75, 8.0, 8.25, 8.5, 8.75, 9.0, 11.75, -16.75, 4.75, 5.0, 5.25, 5.5, 5.75, 6.0, 6.25, 6.5, 6.75, 8.5, 8.75, 9.0, 12.0, 4.75, 5.0, 5.25, 5.5, 5.75, 6.75, 7.5, 9.0, 10.25, 10.5, 11.0, 11.25, 12.0, 4.75, 5.0, 5.25, 5.5, 5.75, 6.75, 7.0, 7.5, 10.0, 10.25, 10.5, 10.75, 11.0, 11.25, 11.5, 11.75, 12.0, 12.25, -11.75, 4.75, 5.0, 5.25, 5.5, 5.75, 6.5, 6.75, 7.5, 10.0, 10.25, 10.5, 10.75, 11.0, 11.25, 11.5, 11.75, 12.0, -14.0, -12.0, 4.75, 5.0, 5.25, 5.5, 5.75, 6.0, 6.5, 7.25, 7.5, 9.75, 10.0, 10.25, 10.5, 10.75, 11.0, 11.25, 11.5, -14.0, -13.75, -13.5, -10.5, 4.75, 5.0, 5.25, 5.5, 5.75, 6.0, 6.25, 6.5, 7.0, 7.25, 10.0, 10.25, 10.5, 10.75, 11.0, 11.25, 11.5, -14.0, -13.5, -10.75, -10.25, -10.0, 5.5, 6.0, 6.5, 6.75, 7.0, 7.25, 10.25, 10.5, 10.75, 11.5, -10.5, -10.25, -10.0, -9.75, 6.5, 6.75, 7.0, 10.0, 10.25, 10.5, 10.75, 11.0, 11.5, -10.25, -10.0, -9.5, -9.25, -8.5, 6.5, 7.25, 7.5, 7.75, 10.0, 10.25, 10.75, 11.0, 11.25, 11.5, -9.75, -9.5, -9.0, -8.75, -8.5, -8.25, 7.25, 10.75, 11.0, 11.25, 11.75, -9.25, -8.75, -8.5, -8.25, -8.0, 10.5, 10.75, 11.0, 11.25, 12.0, -9.0, -8.5, -8.25, -8.0, -7.75, 10.75, 11.0, 41.25, 41.5, -8.75, -8.25, -8.0, -7.75, -7.5, -7.25, -6.75, 8.75, 9.0, 11.0, 41.25, -10.25, -8.0, -7.75, -7.25, -7.0, -6.75, -6.5, 8.5, 8.75, 9.0, -10.5, -7.5, -6.75, -6.5, -6.25, 2.75, 3.0, 3.5, 3.75, 8.5, 8.75, 9.0, -7.0, -6.5, -6.25, -6.0, 2.75, 3.0, 3.25, 3.5, 4.25, 8.25, 8.5, 8.75, 9.0, 9.75, 10.0, -6.75, -6.25, -6.0, -5.75, -5.5, 2.25, 2.5, 2.75, 3.0, 3.25, 3.5, 3.75, 4.0, 4.25, 8.0, 8.25, 8.5, 8.75, 9.0, 9.5, 9.75, 10.0, 10.25, -6.5, -6.25, -5.75, -5.5, -5.25, 2.5, 2.75, 3.0, 3.25, 3.5, 3.75, 4.0, 4.25, 4.5, 4.75, 5.0, 7.75, 8.0, 8.25, 8.5, 8.75, 9.0, 9.25, 9.5, 9.75, 10.0, -6.0, -5.75, -5.5, -5.25, 2.25, 2.5, 2.75, 3.25, 3.5, 3.75, 4.25, 4.5, 4.75, 5.0, 5.5, 5.75, 7.5, 7.75, 8.0, 8.25, 8.75, 9.0, 9.25, 9.75, 10.0, -6.0, -5.5, 2.5, 3.0, 3.25, 4.5, 4.75, 5.0, 5.25, 5.5, 7.75, 8.75, 9.0, 9.25, -23.0, -22.75, -7.25, -7.0, -5.75, -5.5, 2.25, 2.5, 2.75, 3.0, 4.5, 4.75, 5.0, 5.25, 5.5, 5.75, 6.5, 8.5, 8.75, 9.0, 9.25, 9.5, -7.25, -5.75, -5.5, 2.5, 2.75, 5.0, 5.75, 6.0, 6.25, 6.5, 6.75, 8.25, 8.5, 8.75, 9.0, 9.25, 9.5, -5.5, -4.25, -4.0, -3.75, 3.5, 5.75, 6.0, 6.25, 6.5, 7.5, 8.25, 8.5, 8.75, 9.0, 9.25, 9.5, 9.75, -6.0, -4.0, -3.75, 3.5, 3.75, 4.0, 5.5, 5.75, 6.5, 7.25, 8.75, 9.0, 9.25, 9.5, 9.75, -6.25, -6.0, -3.75, -3.5, 7.0, 7.25, 7.5, 7.75, 8.75, 9.0, 9.25, 9.5, 10.0, -6.0, -3.0, -2.75, -2.5, 7.0, 7.25, 7.5, 8.5, 8.75, 9.0, 9.25, 9.5, 9.75, 10.0, -2.75, -2.5, 7.5, 8.5, 8.75, 9.0, 9.25, 9.5, 7.25, 8.25, 8.5, 8.75, 9.0, 9.25, 9.5, -1.5, -1.25, 0.0, 7.0, 7.25, 8.25, 8.5, 8.75, 9.0, -1.25, -1.0, 0.25, 0.5, 0.75, 6.75, 7.0, 7.75, 8.0, 8.25, 8.75, 9.0, -1.5, -1.25, -0.25, 0.0, 0.25, 0.5, 0.75, 1.0, 1.25, 6.25, 6.5, 7.0, 7.75, 8.25, 8.5, -2.0, -1.25, -1.0, -0.5, 0.25, 0.5, 0.75, 1.0, 1.25, 1.5, 1.75, 2.0, 2.25, 6.25, 6.5, 6.75, 7.0, 7.25, 8.0, 8.25, 8.5, -1.75, 0.0, 0.25, 1.25, 1.5, 1.75, 2.0, 6.25, 6.5, 6.75, 7.0, 8.25, 20.5, 20.75, 6.5, 7.75, 8.0, 8.25, 20.75, 2.5, 7.75, 8.0, 9.25, 24.0, -0.75, 2.25, 3.0, 3.25, 3.5, 6.25, 7.75, 8.25, 8.5, 9.0, 9.25, 24.0, -1.0, -0.75, -0.5, 2.75, 3.0, 3.25, 6.25, 6.5, 8.0, 23.25, 24.0, 24.25, -0.5, -0.25, 6.75, 7.0, 23.25, 23.5, 23.75, 24.0, 24.75, 6.0, 6.25, 23.5, 24.0, 24.25, 24.75, 25.0, 5.75, 6.0, 6.25, 23.0, 23.25, 23.5, 23.75, 24.0, 25.0, 23.25, 23.5, 23.75, 24.0, 24.25, -17.5, 6.25, 23.25, 23.5, -18.0, -17.75, -13.0, -12.75, 6.5, 21.25, 23.0, 23.25, 23.5, -22.25, -22.0, -17.75, -13.25, -13.0, -12.75, 2.25, 2.5, 21.0, 21.25, 22.5, 22.75, 23.0, 23.5, -22.25, -22.0, -17.75, -12.75, 2.25, 20.75, 21.0, 22.5, 22.75, 23.0, 23.25, 22.5, 23.0, 22.75, 23.0, 22.75, -8.25, -8.25, -8.0, -7.75, -8.5, -8.25, -8.0, -8.5, -12.25, -12.0, -12.25, -12.0, -5.5, -5.25, -5.0, -5.75, -5.5, -5.25, -5.0, -1.0, -0.75, -1.0, 0.75, 1.25, 0.75, 1.0, 1.25, 1.75, 2.75, 3.0, 3.25, 1.75, 2.0, 2.25, 2.5, 2.75, 3.0, 3.25, 4.5, 4.75, 6.0, 6.25, 2.0, 2.25, 2.5, 2.75, 3.5, 3.75, 4.5, 5.0, 5.25, 5.5, 5.75, 6.0, 2.5, 2.75, 3.5, 5.25, 5.5, 5.75, 5.5, 5.75, 7.25, 5.25, 5.5, 7.5]}, {"Y"=[], "Y"=[]}, {"Y"=[4.403267718525607, -0.3834138109836136, -1.5800841933609058, -2.7767545757381975, -9.560074837456723, -19.300558232052914], "Y"=[20.53747853336786, 11.757519539439958, 9.562529790957988, 7.367540042476016, 5.370901310266658, 3.1075004974198963]}]
  out "obs":dbl[][](array[numeric])=[[2.25, 8.0], [2.25, 8.75], [2.25, 9.0], [2.5, 8.0], [2.5, 8.25], [2.5, 8.5], [2.5, 8.75], [2.5, 9.0], [2.75, 7.75], [2.75, 8.0], [2.75, 8.25], [2.75, 8.5], [2.75, 8.75], [2.75, 9.0], [3.0, 7.75], [3.0, 8.0], [3.0, 8.25], [3.0, 8.5], [3.0, 8.75], [3.0, 9.0], [3.25, 7.5], [3.25, 7.75], [3.25, 8.0], [3.25, 8.25], [3.25, 8.5], [3.5, 0.0], [3.5, 0.25], [3.5, 0.5], [3.5, 0.75], [3.5, 1.0], [3.5, 1.25], [3.5, 1.5], [3.5, 1.75], [3.5, 7.5], [3.5, 7.75], [3.5, 8.0], [3.5, 8.5], [3.75, -2.0], [3.75, -1.75], [3.75, -1.5], [3.75, -1.25], [3.75, -1.0], [3.75, -0.75], [3.75, -0.25], [3.75, 0.0], [3.75, 0.25], [3.75, 0.5], [3.75, 0.75], [3.75, 1.0], [3.75, 1.25], [3.75, 1.5], [3.75, 1.75], [3.75, 7.5], [3.75, 7.75], [4.0, -2.0], [4.0, -1.75], [4.0, -1.5], [4.0, -1.25], [4.0, -1.0], [4.0, -0.75], [4.0, -0.5], [4.0, -0.25], [4.0, 0.0], [4.0, 0.25], [4.0, 0.5], [4.0, 0.75], [4.0, 1.0], [4.0, 1.25], [4.0, 1.5], [4.0, 1.75], [4.0, 7.75], [4.0, 8.0], [4.0, 8.25], [4.0, 8.5], [4.0, 9.0], [4.0, 9.25], [4.25, -2.0], [4.25, -1.75], [4.25, -1.5], [4.25, -1.25], [4.25, -1.0], [4.25, -0.75], [4.25, -0.5], [4.25, -0.25], [4.25, 0.0], [4.25, 0.25], [4.25, 0.5], [4.25, 0.75], [4.25, 1.0], [4.25, 1.25], [4.25, 1.5], [4.25, 1.75], [4.25, 2.0], [4.25, 7.75], [4.25, 8.0], [4.25, 8.25], [4.25, 8.5], [4.25, 9.25], [4.5, -2.0], [4.5, -1.75], [4.5, -1.5], [4.5, -1.25], [4.5, -1.0], [4.5, -0.75], [4.5, -0.5], [4.5, -0.25], [4.5, 0.0], [4.5, 0.25], [4.5, 0.5], [4.5, 0.75], [4.5, 1.0], [4.5, 1.25], [4.5, 1.5], [4.5, 1.75], [4.5, 2.0], [4.5, 7.75], [4.5, 8.0], [4.5, 8.25], [4.75, -2.0], [4.75, -1.75], [4.75, -1.5], [4.75, -1.25], [4.75, -1.0], [4.75, -0.75], [4.75, -0.5], [4.75, 0.0], [4.75, 0.25], [4.75, 0.5], [4.75, 1.0], [4.75, 1.25], [4.75, 1.5], [4.75, 1.75], [4.75, 2.0], [4.75, 7.5], [4.75, 7.75], [4.75, 8.0], [4.75, 8.25], [4.75, 8.5], [4.75, 9.0], [5.0, -2.0], [5.0, -0.75], [5.0, -0.5], [5.0, -0.25], [5.0, 0.0], [5.0, 0.25], [5.0, 0.5], [5.0, 0.75], [5.0, 1.0], [5.0, 1.25], [5.0, 1.5], [5.0, 1.75], [5.0, 2.0], [5.0, 7.5], [5.0, 7.75], [5.0, 8.0], [5.0, 8.25], [5.0, 9.25], [5.25, -2.0], [5.25, -0.75], [5.25, -0.5], [5.25, -0.25], [5.25, 0.25], [5.25, 0.5], [5.25, 1.75], [5.25, 7.5], [5.25, 8.0], [5.25, 8.25], [5.5, -2.0], [5.5, -1.0], [5.5, -0.75], [5.5, -0.5], [5.5, -0.25], [5.5, 1.75], [5.5, 2.0], [5.5, 8.0], [5.5, 8.25], [5.5, 8.5], [5.75, -2.0], [5.75, -1.75], [5.75, -1.0], [5.75, -0.75], [5.75, -0.5], [5.75, -0.25], [5.75, 0.25], [5.75, 0.5], [5.75, 1.5], [5.75, 1.75], [5.75, 8.0], [5.75, 8.25], [5.75, 8.5], [5.75, 9.5]]
  out "lane":dbl[][](array[numeric])=[[2.25, 6.5], [2.25, 7.25], [2.5, 4.5], [2.5, 5.0], [2.5, 5.25], [2.5, 5.5], [2.5, 6.0], [2.5, 6.5], [2.5, 7.25], [2.75, 2.75], [2.75, 3.0], [2.75, 3.25], [2.75, 3.5], [2.75, 3.75], [2.75, 4.0], [2.75, 4.5], [2.75, 4.75], [2.75, 5.0], [2.75, 5.25], [2.75, 7.0], [3.0, 2.75], [3.0, 3.0], [3.0, 3.25], [3.0, 3.5], [3.0, 4.5], [3.0, 4.75], [3.5, 4.75], [3.75, 7.25], [4.0, 4.75], [4.0, 5.0], [4.0, 7.25], [4.5, 5.0], [4.75, 4.75], [4.75, 5.0], [5.25, 5.0], [5.5, 5.0], [6.0, 5.25], [6.25, 5.0], [6.25, 5.25], [6.75, 4.75], [7.0, 2.75], [7.0, 5.25], [7.0, 5.5], [7.25, 4.5], [7.5, 6.0]]
  in  "y_min":dbl=1.0
  in  "y_max":dbl=10.0
  out "x_max":dbl=6.0
  out "x_min":dbl=1.0
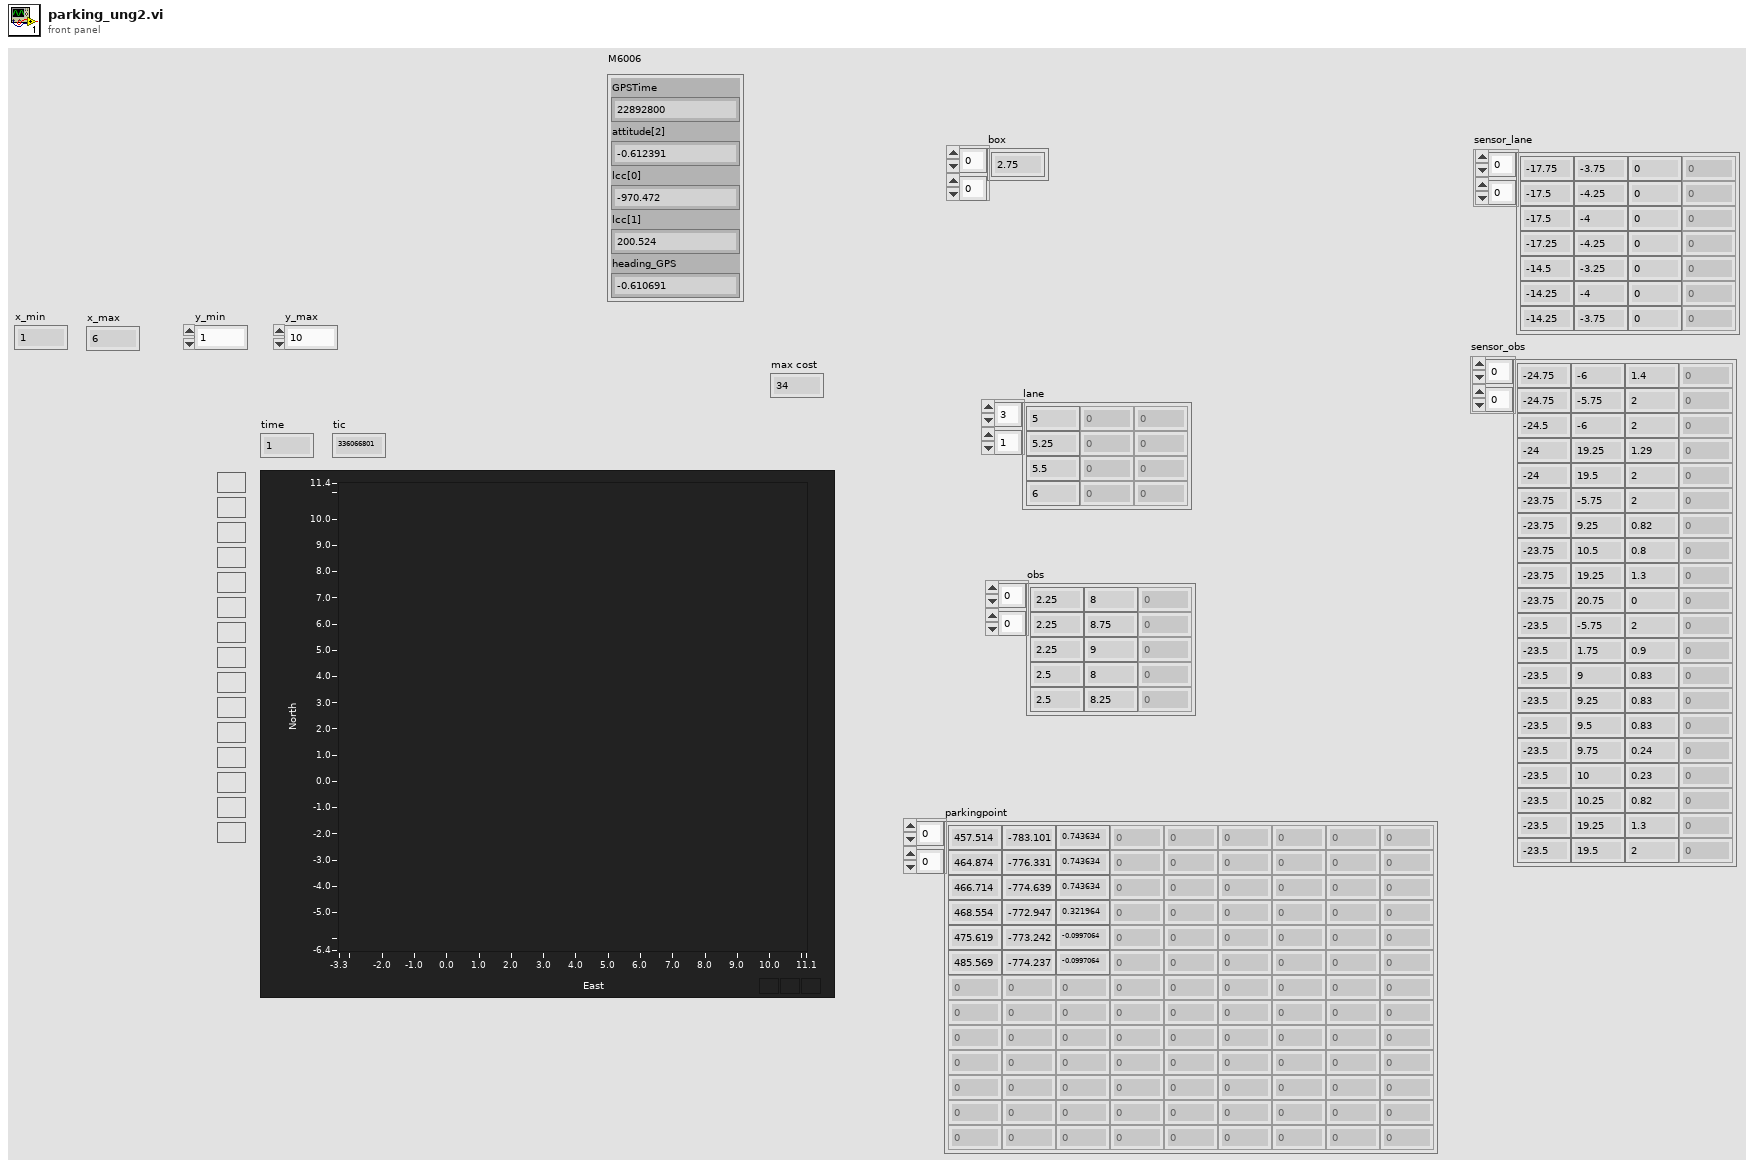
[diagram p1: front panel]
types:
  T1 = cluster{"GPSTime":dbl, "attitude[2]":sgl, "lcc[0]":sgl, "lcc[1]":sgl, "heading_GPS":sgl}
  T2 = cluster{"GPSTime":dbl, "attitude[2]":dbl, "lcc[0]":dbl, "lcc[1]":dbl, "heading_GPS":dbl}
  T3 = cluster{"idx":i32, "x":dbl, "y":dbl, "h":dbl, "x_path":dbl}
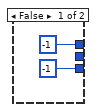
[diagram p3: hidden frame]
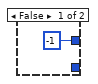
[diagram p4: hidden frame]
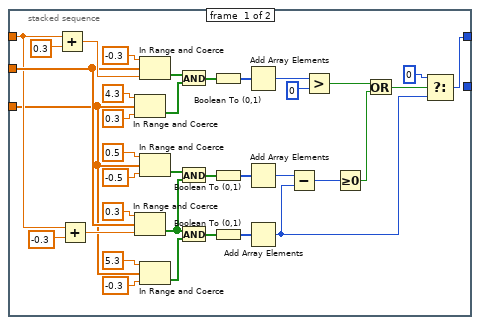
[diagram p5: hidden frame]
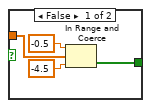
[diagram p7: hidden frame]
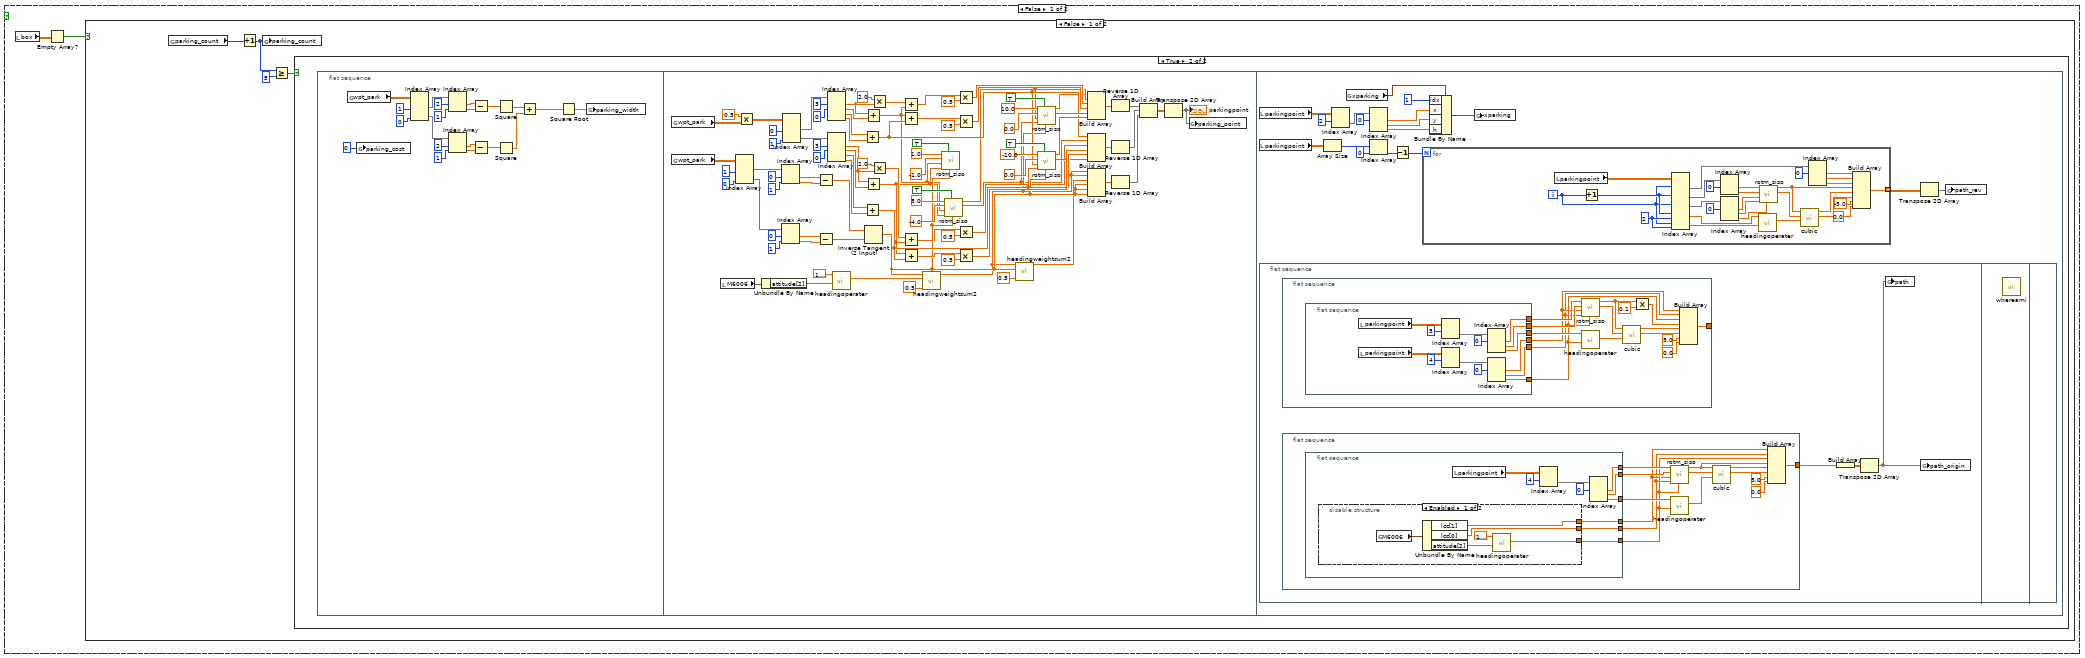
[diagram p8: hidden frame]
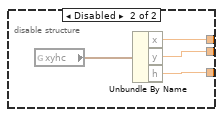
[diagram p10: hidden frame]
diagram:
  n1 = flat-sequence {
    tunnel: [w637] -> w2
    tunnel: [w636] -> w1
    tunnel: w2 -> [w651]
    tunnel: w1 -> [w650]
    frame #0 {
      n2 = flat-sequence {
        frame #0 {
        }
      }
      n3 = Tick Count (ms)() -> (millisecond timer value=→"tic":u32)
      n4 = global read "G_SEN.vi" "sensor_lane"() -> (→"sensor_lane":dbl[][])
      n5 = global read "G_SEN.vi" "sensor_obs"() -> (→"sensor_obs":dbl[][])
      n6 = global read "G_NAV.vi" "M6006"() -> (→"M6006":T2)
    }
    frame #1 {
      n7 = local read "sensor_lane"() -> (w7:dbl[][])
      n8 = Index Array(array=w7, index (col) #1=0 ("disabled index (col)"), index (col) #2=1 ("index (col)")) -> (element #1=w20:dbl[], element #2=w19:dbl[])  [unwired: 2 in]
      n9 = local read "y_max"() -> (w27:dbl)
      n10 = local read "y_min"() -> (w28:dbl)
      n11 = Greater Or Equal To 0?(x=w20) -> (x >= 0?=w21:bool[])
      n12 = In Range and Coerce(upper limit=w27, x=w19, lower limit=w28) -> (In Range?=w26:bool[])  [unwired: 1 out]
      n13 = And(x=w21, y=w26) -> (x .and. y?=w25:bool[])
      n14 = Boolean To (0,1)(Boolean=w25) -> (0, 1=w24:i16[])
      n15 = Build Cluster Array(w24, w20) -> (w23:cluster{i16, "element":dbl}[])
      n16 = Sort 1D Array(array=w23) -> (sorted array=w22:cluster{i16, "element":dbl}[])
      n17 = for {
        tunnel: w22 -> [w33] mode=indexing
        tunnel: [w32] -> w18 mode=indexing
        tunnel: [w31] -> w17 mode=indexing
        n18 = Unbundle(w33) -> (w32:i16, "element"=w31:dbl)
      }
      n19 = Add Array Elements(numeric array=w18) -> (sum=w15:i16)
      n20 = Array Max & Min(array=w18) -> (max index (indices)=w16:i32)  [unwired: 3 out]
      n21 = Array Subset(array=w17, index=w16, length=w15) -> (w14:dbl[])
      n22 = Array Max & Min(array=w14) -> (min value=w11:dbl)  [unwired: 3 out]
      n23 = Decrement(x=w11) -> (x-1=w9:dbl)
      n24 = Add(x=w11, y=4.0) -> (x+y=→"x_max":dbl)
      n25 = Max & Min(x=1.0, y=w9) -> (max(x,y)=→"x_min":dbl)  [unwired: 1 out]
    }
    frame #2 {
      n26 = local read "sensor_obs"() -> (w34:dbl[][])
      n27 = Index Array(array=w34, index (col) #1=0 ("disabled index (col)"), index (col) #2=1 ("index (col)")) -> (element #1=w44:dbl[], element #2=w45:dbl[])  [unwired: 2 in]
      n28 = local read "x_max"() -> (w37:dbl)
      n29 = local read "y_max"() -> (w40:dbl)
      n30 = local read "y_min"() -> (w39:dbl)
      n31 = local read "x_min"() -> (w38:dbl)
      n32 = In Range and Coerce(upper limit=w37, x=w44, lower limit=w38) -> (In Range?=w42:bool[])  [unwired: 1 out]
      n33 = In Range and Coerce(upper limit=w40, x=w45, lower limit=w39) -> (In Range?=w41:bool[])  [unwired: 1 out]
      n34 = And(x=w42, y=w41) -> (x .and. y?=w43:bool[])
      n35 = Boolean To (0,1)(Boolean=w43) -> (0, 1=w46:i16[])
      n36 = Build Cluster Array(w46, w44, w45) -> (w47:cluster{i16, "element":dbl, "element":dbl}[])
      n37 = Sort 1D Array(array=w47) -> (sorted array=w48:cluster{i16, "element":dbl, "element":dbl}[])
      n38 = for {
        tunnel: w48 -> [w61] mode=indexing
        tunnel: [w60] -> w49 mode=indexing
        tunnel: [w59] -> w50 mode=indexing
        tunnel: [w58] -> w53 mode=indexing
        n39 = Unbundle(w61) -> (w60:i16, "element"=w59:dbl, "element"=w58:dbl)
      }
      n40 = Add Array Elements(numeric array=w49) -> (sum=w52:i16)
      n41 = Array Max & Min(array=w49) -> (max index (indices)=w51:i32)  [unwired: 3 out]
      n42 = Array Subset(array=w50, index=w51, length=w52) -> (w54:dbl[])
      n43 = Array Subset(array=w53, index=w51, length=w52) -> (w55:dbl[])
      n44 = Build Array(w54, w55) -> (w56:dbl[][])
      n45 = Transpose 2D Array(2D array=w56) -> (transposed array=→"obs":dbl[][])
    }
    frame #3 {
      n46 = local read "y_max"() -> (w75:dbl)
      n47 = local read "y_min"() -> (w74:dbl)
      n48 = local read "obs"() -> (w81:dbl[][])
      n49 = Subtract(x=w75, y=w74) -> (x-y=w73:dbl)
      n50 = Index Array(array=w81, index (col)=1 ("disabled index (col)")) -> (element=w79:dbl[])  [unwired: 1 in]
      n51 = Sort 1D Array(array=w79) -> (sorted array=w78:dbl[])
      n52 = Divide(x=w73, y=0.1 ("step")) -> (x/y=w71:dbl)
      n53 = local read "y_min"() -> (w77:dbl)
      n54 = call "histung.vi"("size"=w71, "cropresult"=FALSE, "step"=0.1, "start"=w77, "X"=w78) -> ("H(x)"=w69:i32[])  [unwired: 5 in, 1 out]
      n55 = for {
        tunnel: w69 -> [w127] mode=indexing
        shift-right: [w122] -> _
        shift-left: i16 0 -> [w125]
        tunnel: [w122] -> w67 mode=indexing
        n56 = Increment(x=w125) -> (x+1=w124:i16)
        n57 = Equal To 0?(x=w127) -> (x = 0?=w126:bool)
        n58 = Select(t=w124, s=w126, f=i16 0) -> (s? t:f=w122:i16)
      }
      n59 = Array Max & Min(array=w67) -> (max value=w63:i16, max index (indices)=w64:i32)  [unwired: 2 out]
      n60 = Greater Or Equal?(x=w63, y=i16 20) -> (x >= y?=w65:bool)
      n61 = case shown="True" w65 {
        tunnel: w64 -> [_ w109]
        tunnel: w63 -> [_ w117]
        tunnel: [_ w86] -> w62
        frame False {
        }
        frame True {
          n62 = Subtract(x=w109, y=w117) -> (x-y=w116:i32)
          n63 = Increment(x=w116) -> (x+1=w114:i32)
          n64 = local read "sensor_lane"() -> (w82:dbl[][])
          n65 = local read "x_max"() -> (w84:dbl)
          n66 = Multiply(x=w109, y=0.1 ("step")) -> (x*y=w108:dbl)
          n67 = Multiply(x=w114, y=0.1 ("step")) -> (x*y=w113:dbl)
          n68 = local read "y_min"() -> (w111:dbl)
          n69 = local read "y_min"() -> (w112:dbl)
          n70 = Add(x=2.0, y=w84) -> (x+y=w85:dbl)
          n71 = Index Array(array=w82, index (col) #1=0 ("disabled index (col)"), index (col) #2=1 ("index (col)")) -> (element #1=w101:dbl[], element #2=w100:dbl[])  [unwired: 2 in]
          n72 = local read "x_min"() -> (w105:dbl)
          n73 = Add(x=w108, y=w111) -> (x+y=w87:dbl)
          n74 = Add(x=w113, y=w112) -> (x+y=w88:dbl)
          n75 = In Range and Coerce(upper limit=w85, x=w101, lower limit=w105) -> (In Range?=w103:bool[])  [unwired: 1 out]
          n76 = In Range and Coerce(upper limit=w87, x=w100, lower limit=w88) -> (In Range?=w104:bool[])  [unwired: 1 out]
          n77 = And(x=w103, y=w104) -> (x .and. y?=w102:bool[])
          n78 = Boolean To (0,1)(Boolean=w102) -> (0, 1=w99:i16[])
          n79 = Build Cluster Array(w99, w101, w100) -> (w98:cluster{i16, "element":dbl, "element":dbl}[])
          n80 = Sort 1D Array(array=w98) -> (sorted array=w97:cluster{i16, "element":dbl, "element":dbl}[])
          n81 = for {
            tunnel: w97 -> [w121] mode=indexing
            tunnel: [w120] -> w96 mode=indexing
            tunnel: [w119] -> w95 mode=indexing
            tunnel: [w118] -> w92 mode=indexing
            n82 = Unbundle(w121) -> (w120:i16, "element"=w119:dbl, "element"=w118:dbl)
          }
          n83 = Add Array Elements(numeric array=w96) -> (sum=w93:i16)
          n84 = Array Max & Min(array=w96) -> (max index (indices)=w94:i32)  [unwired: 3 out]
          n85 = Array Subset(array=w95, index=w94, length=w93) -> (w91:dbl[])
          n86 = Array Subset(array=w92, index=w94, length=w93) -> (w90:dbl[])
          n87 = Build Array(w91, w90) -> (w89:dbl[][])
          n88 = Transpose 2D Array(2D array=w89) -> (transposed array=w86:dbl[][])
        }
      }
      "lane" <- w62
    }
    frame #4 {
      n89 = flat-sequence {
        tunnel: [w133] -> w130
        tunnel: [w132] -> w129
        tunnel: [w131] -> w128
        tunnel: w130 -> [w272]
        tunnel: w129 -> [w280]
        tunnel: w128 -> [w273]
        frame #0 {
          n90 = local read "lane"() -> (w137:dbl[][])
          n91 = Index Array(array=w137, index (col) #1=1 ("disabled index (col)"), index (col) #2=0 ("index (col)")) -> (element #1=w136:dbl[], element #2=w135:dbl[])  [unwired: 2 in]
          n92 = for {
            tunnel: w136 -> [w161] mode=indexing
            tunnel: w135 -> [w159]
            tunnel: w136 -> [w160]
            tunnel: w135 -> [w158] mode=indexing
            tunnel: [w148] -> w133 mode=indexing
            tunnel: [w147] -> w131 mode=indexing
            tunnel: [w146] -> w132 mode=indexing
            n93 = Subtract(x=w160, y=w161) -> (x-y=w152:dbl[])
            n94 = Subtract(x=w159, y=w158) -> (x-y=w151:dbl[])
            n95 = Square(x=w152) -> (x^2=w157:dbl[])
            n96 = Square(x=w151) -> (x^2=w156:dbl[])
            n97 = Inverse Tangent (2 Input)(1:w151, 2:w152) -> (0:w145:dbl[])
            n98 = Add(x=w157, y=w156) -> (x+y=w150:dbl[])
            n99 = Absolute Value(x=w145) -> (abs(x)=w144:dbl[])
            n100 = Square Root(x=w150) -> (sqrt(x)=w149:dbl[])
            n101 = In Range and Coerce(upper limit=1.75, x=w144, lower limit=0.75) -> (In Range?=w139:bool[])  [unwired: 1 out]
            n102 = In Range and Coerce(upper limit=3.0, x=w149, lower limit=2.0) -> (In Range?=w140:bool[])  [unwired: 1 out]
            n103 = And(x=w140, y=w139) -> (x .and. y?=w141:bool[])
            n104 = Or Array Elements(Boolean array=w141) -> (logical OR=w155:bool)
            n105 = case shown="True" w155 {
              tunnel: w141 -> [_ w176]
              tunnel: w152 -> [_ w175]
              tunnel: w151 -> [_ w174]
              tunnel: w145 -> [_ w173]
              tunnel: w149 -> [_ w166]
              tunnel: [_ w168] -> w148
              tunnel: [-1 ("element") w172] -> w147
              tunnel: [-1 ("element") w169] -> w146
              frame False {
              }
              frame True {
                n106 = Negate(x=w166) -> (-x=w165:dbl[])
                n107 = for {
                  tunnel: w176 -> [w184] mode=indexing
                  tunnel: w175 -> [w183]
                  tunnel: w174 -> [w182]
                  tunnel: w173 -> [w181] mode=indexing
                  tunnel: w165 -> [w180] mode=indexing
                  tunnel: [w179] -> w171 mode=indexing
                  tunnel: [w178] -> w170 mode=indexing
                  tunnel: [w177] -> w164 mode=indexing
                  i -> [w178]
                  n108 = case shown="True" w184 {
                    tunnel: w183 -> [_ w198]
                    tunnel: w182 -> [_ w197]
                    tunnel: w181 -> [_ w195]
                    tunnel: w180 -> [_ w191]
                    tunnel: [-1 w186] -> w179
                    tunnel: [_ w187] -> w177
                    frame False {
                    }
                    frame True {
                      w196 = 0.0 ("y0")
                      n109 = call "rotm_mimo.vi"("angle[rad]"=w195, "y0"=w196, "x0"=w196, "y"=w198, "x"=w197) -> ("Y"=w193:dbl[], "X"=w194:dbl[])  [unwired: 3 in, 2 out]
                      n110 = Negate(x=w194) -> (-x=w192:dbl[])
                      n111 = stacked-sequence {
                        tunnel: w193 -> [w211 w248]
                        tunnel: w192 -> [w217 w253]
                        tunnel: w191 -> [w216 w252]
                        tunnel: [w214 _] -> w190
                        tunnel: [_ w237] -> w189
                        frame #0 {
                          n112 = Add(x=w216, y=0.3) -> (x+y=w222:dbl)
                          n113 = Add(x=w216, y=-0.3) -> (x+y=w230:dbl)
                          n114 = In Range and Coerce(upper limit=4.3, x=w211, lower limit=0.3) -> (In Range?=w224:bool[])  [unwired: 1 out]
                          n115 = In Range and Coerce(upper limit=0.3, x=w217, lower limit=w230) -> (In Range?=w209:bool[])  [unwired: 1 out]
                          n116 = In Range and Coerce(upper limit=-0.3, x=w217, lower limit=w222) -> (In Range?=w223:bool[])  [unwired: 1 out]
                          n117 = In Range and Coerce(upper limit=0.5, x=w211, lower limit=-0.5) -> (In Range?=w210:bool[])  [unwired: 1 out]
                          n118 = In Range and Coerce(upper limit=5.3, x=w211, lower limit=-0.3) -> (In Range?=w229:bool[])  [unwired: 1 out]
                          n119 = And(x=w223, y=w224) -> (x .and. y?=w225:bool[])
                          n120 = And(x=w210, y=w209) -> (x .and. y?=w207:bool[])
                          n121 = And(x=w209, y=w229) -> (x .and. y?=w228:bool[])
                          n122 = Boolean To (0,1)(Boolean=w225) -> (0, 1=w226:i16[])
                          n123 = Boolean To (0,1)(Boolean=w207) -> (0, 1=w208:i16[])
                          n124 = Boolean To (0,1)(Boolean=w228) -> (0, 1=w227:i16[])
                          n125 = Add Array Elements(numeric array=w226) -> (sum=w200:i16)
                          n126 = Add Array Elements(numeric array=w208) -> (sum=w206:i16)
                          n127 = Add Array Elements(numeric array=w227) -> (sum=w205:i16)
                          n128 = Subtract(x=w206, y=w205) -> (x-y=w204:i16)
                          n129 = Greater?(x=w200, y=i16 0) -> (0:w203:bool)
                          n130 = Greater Or Equal To 0?(x=w204) -> (x >= 0?=w202:bool)
                          n131 = Or(x=w203, y=w202) -> (x .or. y?=w201:bool)
                          n132 = Select(t=i16 0, s=w201, f=w205) -> (s? t:f=w214:i16)
                        }
                        frame #1 {
                          n133 = Add(x=w252, y=0.3) -> (x+y=w258:dbl)
                          n134 = Add(x=w252, y=-0.3) -> (x+y=w266:dbl)
                          n135 = In Range and Coerce(upper limit=0.3, x=w253, lower limit=w266) -> (In Range?=w246:bool[])  [unwired: 1 out]
                          n136 = In Range and Coerce(upper limit=-0.3, x=w253, lower limit=w258) -> (In Range?=w259:bool[])  [unwired: 1 out]
                          n137 = In Range and Coerce(upper limit=-0.3, x=w248, lower limit=-4.3) -> (In Range?=w260:bool[])  [unwired: 1 out]
                          n138 = In Range and Coerce(upper limit=0.5, x=w248, lower limit=-0.5) -> (In Range?=w247:bool[])  [unwired: 1 out]
                          n139 = In Range and Coerce(upper limit=0.3, x=w248, lower limit=-5.3) -> (In Range?=w265:bool[])  [unwired: 1 out]
                          n140 = And(x=w259, y=w260) -> (x .and. y?=w261:bool[])
                          n141 = And(x=w247, y=w246) -> (x .and. y?=w244:bool[])
                          n142 = And(x=w246, y=w265) -> (x .and. y?=w264:bool[])
                          n143 = Boolean To (0,1)(Boolean=w261) -> (0, 1=w262:i16[])
                          n144 = Boolean To (0,1)(Boolean=w244) -> (0, 1=w245:i16[])
                          n145 = Boolean To (0,1)(Boolean=w264) -> (0, 1=w263:i16[])
                          n146 = Add Array Elements(numeric array=w262) -> (sum=w236:i16)
                          n147 = Add Array Elements(numeric array=w245) -> (sum=w243:i16)
                          n148 = Add Array Elements(numeric array=w263) -> (sum=w242:i16)
                          n149 = Subtract(x=w243, y=w242) -> (x-y=w241:i16)
                          n150 = Greater?(x=w236, y=i16 0) -> (0:w240:bool)
                          n151 = Greater Or Equal To 0?(x=w241) -> (x >= 0?=w239:bool)
                          n152 = Or(x=w240, y=w239) -> (x .or. y?=w238:bool)
                          n153 = Select(t=i16 0, s=w238, f=w242) -> (s? t:f=w237:i16)
                        }
                      }
                      n154 = Build Array(w190, w189) -> (w188:i16[])
                      n155 = Array Max & Min(array=w188) -> (max value=w187:i16, max index (indices)=w186:i32)  [unwired: 2 out]
                    }
                  }
                }
                n156 = Array Max & Min(array=w164) -> (max value=w168:i16, max index (indices)=w167:i32)  [unwired: 2 out]
                n157 = Index Array(array=w171, index=w167) -> (element=w172:i32)
                n158 = Index Array(array=w170, index=w167) -> (element=w169:i32)
              }
            }
          }
        }
        frame #1 {
          n159 = Array Max & Min(array=w272) -> (max value=w274:i16, max index (indices)=w276:i32)  [unwired: 2 out]
          "max cost" <- w274
          n160 = Index Array(array=w273, index=w276) -> (element=w278:i32)
          n161 = Index Array(array=w280, index=w276) -> (element=w277:i32)
          n162 = Greater Or Equal?(x=w274, y=i16 20) -> (x >= y?=w271:bool)
          n163 = case shown="True" w271 {
            tunnel: w277 -> [_ w325]
            tunnel: w276 -> [_ w324]
            tunnel: w278 -> [_ w298]
            tunnel: [_ w295] -> w275
            tunnel: w274 -> [_ _]
            frame False {
            }
            frame True {
              w307 = 0.0 ("element")
              w303 = dbl[] [0.0, 5.0, 5.0, 0.0, 0.0]
              n164 = local read "lane"() -> (w326:dbl[][])
              n165 = Index Array(array=w326, index (row) #1=w325, index (row) #2=w324) -> (element #1=w323:dbl[], element #2=w317:dbl[])  [unwired: 2 in]
              n166 = Subtract(x=w323, y=w317) -> (x-y=w311:dbl[])
              n167 = Index Array(array=w317, index #1=0 ("index")) -> (element #1=w301:dbl, element #2=w300:dbl)  [unwired: 1 in]
              n168 = Square(x=w311) -> (x^2=w310:dbl[])
              n169 = Index Array(array=w311, index #1=1 ("index"), index #2=0 ("index")) -> (element #1=w320:dbl, element #2=w319:dbl)
              n170 = Add Array Elements(numeric array=w310) -> (sum=w309:dbl)
              n171 = Inverse Tangent (2 Input)(1:w319, 2:w320) -> (0:w313:dbl)
              n172 = Square Root(x=w309) -> (sqrt(x)=w308:dbl)
              n173 = call "headingoperater.vi"("h1"=w313, "h2"=1.5707963267948966) -> ("h2+h1"=w299:dbl)  [unwired: 8 in, 1 out]
              n174 = Equal To 0?(x=w298) -> (x = 0?=w297:bool)
              n175 = Negate(x=w303) -> (-x=w302:dbl[])
              n176 = Negate(x=w308) -> (-x=w296:dbl)
              n177 = flat-sequence {
                tunnel: w301 -> [w341]
                tunnel: w300 -> [w340]
                tunnel: w299 -> [w339]
                tunnel: w297 -> [w336]
                tunnel: w296 -> [w333]
                tunnel: [w327] -> w290
                frame #0 {
                  n178 = local read "sensor_obs"() -> (w346:dbl[][])
                  n179 = Index Array(array=w346, index (col) #1=0 ("disabled index (col)"), index (col) #2=1 ("index (col)")) -> (element #1=w343:dbl[], element #2=w342:dbl[])  [unwired: 2 in]
                  n180 = call "rotm_mimo.vi"("angle[rad]"=w339, "reverse"=FALSE, "y0"=w340, "x0"=w341, "y"=w342, "x"=w343) -> ("Y"=w334:dbl[], "X"=w337:dbl[])  [unwired: 2 in, 2 out]
                  n181 = case shown="True" w336 {
                    tunnel: w337 -> [w349 w354]
                    tunnel: [w347 w351] -> w329
                    frame False {
                      n182 = In Range and Coerce(upper limit=-0.5, x=w349, lower limit=-4.5) -> (In Range?=w347:bool[])  [unwired: 1 out]
                    }
                    frame True {
                      n183 = In Range and Coerce(upper limit=4.5, x=w354, lower limit=0.5) -> (In Range?=w351:bool[])  [unwired: 1 out]
                    }
                  }
                  n184 = Add(x=0.2, y=w333) -> (x+y=w331:dbl)
                  n185 = In Range and Coerce(upper limit=-0.2, x=w334, lower limit=w331) -> (In Range?=w328:bool[])  [unwired: 1 out]
                  n186 = And(x=w328, y=w329) -> (x .and. y?=w330:bool[])
                  n187 = Or Array Elements(Boolean array=w330) -> (logical OR=w327:bool)
                }
              }
              n188 = Select(t=w303, s=w297, f=w302) -> (s? t:f=w304:dbl[])
              n189 = Build Array(w307, w307, w296, w296, 0.0 ("element")) -> (w305:dbl[])
              n190 = call "rotm_mimo.vi"("angle[rad]"=w299, "reverse"=TRUE, "y0"=w300, "x0"=w301, "y"=w305, "x"=w304) -> ("Y"=w315:dbl[], "X"=w288:dbl[])  [unwired: 2 in, 2 out]
              n191 = Build Array(w288, w315) -> (w314:dbl[][])
              n192 = Array Subset(array=w288, length=4) -> (w286:dbl[])  [unwired: 1 in]
              n193 = Add Array Elements(numeric array=w286) -> (sum=w292:dbl)
              n194 = Transpose 2D Array(2D array=w314) -> (transposed array=w294:dbl[][])
              n195 = Multiply(x=0.25, y=w292) -> (x*y=w285:dbl)
              n196 = In Range and Coerce(upper limit=7.0, x=w285, lower limit=3.0) -> (In Range?=w282:bool)  [unwired: 1 out]
              n197 = Not(x=w282) -> (.not. x?=w281:bool)
              n198 = Or(x=w290, y=w281) -> (x .or. y?=w289:bool)
              n199 = Select(t=dbl[][] [], s=w289, f=w294) -> (s? t:f=w295:dbl[][])
            }
          }
          "box" <- w275
        }
        frame #2 {
          n200 = global read "G_PATH.vi" "parking_cost"() -> (w355:i32)
          n201 = local read "box"() -> (w361:dbl[][])
          n202 = local read "max cost"() -> (w360:i32)
          n203 = Empty Array?(array=w361) -> (empty?=w359:bool)
          n204 = Not(x=w359) -> (.not. x?=w358:bool)
          n205 = Greater?(x=w360, y=w355) -> (0:w357:bool)
          n206 = And(x=w358, y=w357) -> (x .and. y?=w356:bool)
          n207 = case shown="True" w356 {
            frame False {
              n208 = local read "box"() -> (w363:dbl[][])
              n209 = Empty Array?(array=w363) -> (empty?=w362:bool)
              n210 = case shown="False" w362 {
                frame False {
                  n211 = global read "G_PATH.vi" "parking_count"() -> (w365:i32)
                  n212 = Increment(x=w365) -> (x+1=w364:i32)
                  n213 = global write "G_PATH.vi" "parking_count"(w364) -> ()
                  n214 = Greater Or Equal?(x=w364, y=5) -> (x >= y?=w366:bool)
                  n215 = case shown="True" w366 {
                    frame False {
                    }
                    frame True {
                      n216 = flat-sequence {
                        frame #0 {
                          n217 = global read "G_PATH.vi" "wpt_park"() -> (w369:dbl[][])
                          n218 = global write "G_PATH.vi" "parking_cost"(0 ("parkingcost")) -> ()
                          n219 = Index Array(array=w369, index (col) #1=1 ("disabled index (col)"), index (col) #2=0 ("index (col)")) -> (element #1=w384:dbl[], element #2=w385:dbl[])  [unwired: 2 in]
                          n220 = Index Array(array=w384, index #1=2 ("index"), index #2=1 ("index")) -> (element #1=w386:dbl, element #2=w372:dbl)
                          n221 = Index Array(array=w385, index #1=2 ("index"), index #2=1 ("index")) -> (element #1=w371:dbl, element #2=w387:dbl)
                          n222 = Subtract(x=w386, y=w372) -> (x-y=w377:dbl)
                          n223 = Subtract(x=w371, y=w387) -> (x-y=w376:dbl)
                          n224 = Square(x=w377) -> (x^2=w375:dbl)
                          n225 = Square(x=w376) -> (x^2=w374:dbl)
                          n226 = Add(x=w375, y=w374) -> (x+y=w373:dbl)
                          n227 = Square Root(x=w373) -> (sqrt(x)=w368:dbl)
                          n228 = global write "G_PATH.vi" "parking_width"(w368) -> ()
                        }
                        frame #1 {
                          n229 = global read "G_PATH.vi" "wpt_park"() -> (w390:dbl[][])
                          n230 = global read "G_PATH.vi" "wpt_park"() -> (w389:dbl[][])
                          n231 = local read "M6006"() -> (w438:T1)
                          n232 = Index Array(array=w389, index (col) #1=1 ("disabled index (col)"), index (col) #2=0 ("index (col)")) -> (element #1=w440:dbl[], element #2=w445:dbl[])  [unwired: 2 in]
                          n233 = Multiply(x=0.5, y=w390) -> (x*y=w468:dbl[][])
                          n234 = Unbundle By Name(w438) -> ("attitude[2]"=w430:sgl)
                          n235 = Index Array(array=w440, index #1=0 ("index"), index #2=1 ("index")) -> (element #1=w448:dbl, element #2=w449:dbl)
                          n236 = Index Array(array=w445, index #1=0 ("index"), index #2=1 ("index")) -> (element #1=w450:dbl, element #2=w451:dbl)
                          n237 = Index Array(array=w468, index (col) #1=0 ("disabled index (col)"), index (col) #2=1 ("index (col)")) -> (element #1=w474:dbl[], element #2=w455:dbl[])  [unwired: 2 in]
                          n238 = Subtract(x=w448, y=w449) -> (x-y=w452:dbl)
                          n239 = Subtract(x=w450, y=w451) -> (x-y=w453:dbl)
                          n240 = Index Array(array=w474, index #1=3 ("index"), index #2=0 ("index")) -> (element #1=w413:dbl, element #2=w471:dbl, element #3=w470:dbl, element #4=w469:dbl)  [unwired: 2 in]
                          n241 = Index Array(array=w455, index #1=3 ("index"), index #2=0 ("index")) -> (element #1=w415:dbl, element #2=w458:dbl, element #3=w459:dbl, element #4=w460:dbl)  [unwired: 2 in]
                          n242 = call "headingoperater.vi"("h1"=w430, "h2"=1.5707963267948966) -> ("h2-h1"=w429:dbl)  [unwired: 8 in, 1 out]
                          n243 = Add(x=w470, y=w469) -> (x+y=w403:dbl)
                          n244 = Add(x=w459, y=w460) -> (x+y=w421:dbl)
                          n245 = Inverse Tangent (2 Input)(1:w453, 2:w452) -> (0:w408:dbl)
                          n246 = Add(x=w413, y=w471) -> (x+y=w402:dbl)
                          n247 = Add(x=w415, y=w458) -> (x+y=w399:dbl)
                          n248 = Multiply(x=2.0, y=w413) -> (x*y=w407:dbl)
                          n249 = Multiply(x=2.0, y=w415) -> (x*y=w401:dbl)
                          n250 = Add(x=w407, y=w402) -> (x+y=w405:dbl)
                          n251 = Add(x=w402, y=w403) -> (x+y=w466:dbl)
                          n252 = Add(x=w401, y=w399) -> (x+y=w398:dbl)
                          n253 = Add(x=w399, y=w421) -> (x+y=w461:dbl)
                          n254 = call "headingweightsum2.vi"("a"=0.5, "h2"=w429, "h1"=w408) -> ("a*h2+(1-a)*h1"=w395:dbl)  [unwired: 8 in]
                          n255 = call "rotm_siso.vi"("angle[rad]"=w408, "reverse"=TRUE, "y0"=w399, "x0"=w402, "y"=-1.0, "x"=1.0) -> ()  [unwired: 4 in, 2 out]
                          n256 = call "rotm_siso.vi"("angle[rad]"=w408, "reverse"=TRUE, "y0"=w399, "x0"=w402, "y"=-4.0, "x"=5.0) -> ("y'"=w392:dbl, "x'"=w394:dbl)  [unwired: 4 in]
                          n257 = Multiply(x=w405, y=0.5) -> (x*y=w404:dbl)
                          n258 = Multiply(x=w466, y=0.5) -> (x*y=w464:dbl)
                          n259 = Multiply(x=w398, y=0.5) -> (x*y=w397:dbl)
                          n260 = Multiply(x=w461, y=0.5) -> (x*y=w463:dbl)
                          n261 = call "headingweightsum2.vi"("a"=0.5, "h2"=w408, "h1"=w395) -> ("a*h2+(1-a)*h1"=w396:dbl)  [unwired: 8 in]
                          n262 = call "rotm_siso.vi"("angle[rad]"=w395, "reverse"=TRUE, "y0"=w392, "x0"=w394, "y"=0.0, "x"=10.0) -> ("y'"=w391:dbl, "x'"=w393:dbl)  [unwired: 4 in]
                          n263 = call "rotm_siso.vi"("angle[rad]"=w408, "reverse"=TRUE, "y0"=w421, "x0"=w403, "y"=0.0, "x"=-10.0) -> ("y'"=w416:dbl, "x'"=w417:dbl)  [unwired: 4 in]
                          n264 = Build Array(w393, w394, w404, w464, w403, w417) -> (w427:dbl[])
                          n265 = Build Array(w391, w392, w397, w463, w421, w416) -> (w425:dbl[])
                          n266 = Build Array(w395, w395, w396, w408, w408, w408) -> (w423:dbl[])
                          n267 = Reverse 1D Array(array=w427) -> (reversed array=w426:dbl[])
                          n268 = Reverse 1D Array(array=w425) -> (reversed array=w424:dbl[])
                          n269 = Reverse 1D Array(array=w423) -> (reversed array=w422:dbl[])
                          n270 = Build Array(w426, w424, w422) -> (w439:dbl[][])
                          n271 = Transpose 2D Array(2D array=w439) -> (transposed array=w388:dbl[][])
                          "parkingpoint" <- w388
                          n272 = global write "G_PATH.vi" "parking_point"(w388) -> ()
                        }
                        frame #2 {
                          n273 = local read "parkingpoint"() -> (w485:dbl[][])
                          n274 = local read "parkingpoint"() -> (w493:dbl[][])
                          n275 = flat-sequence {
                            frame #0 {
                              n276 = flat-sequence {
                                tunnel: [w503] -> _
                                frame #0 {
                                n277 = flat-sequence {
                                tunnel: [w522] -> w506
                                tunnel: [w521] -> w505
                                tunnel: [w520] -> w504
                                tunnel: [w513] -> w502
                                tunnel: [w515] -> w501
                                tunnel: [w514] -> w500
                                frame #0 {
                                n278 = local read "parkingpoint"() -> (w524:dbl[][])
                                n279 = local read "parkingpoint"() -> (w518:dbl[][])
                                n280 = Index Array(array=w524, index (row)=5 ("index")) -> (element=w523:dbl[])  [unwired: 1 in]
                                n281 = Index Array(array=w518, index (row)=4 ("index")) -> (element=w519:dbl[])  [unwired: 1 in]
                                n282 = Index Array(array=w523, index #1=0 ("index")) -> (element #1=w522:dbl, element #2=w521:dbl, element #3=w520:dbl)  [unwired: 2 in]
                                n283 = Index Array(array=w519, index #1=0 ("index")) -> (element #1=w515:dbl, element #2=w514:dbl, element #3=w513:dbl)  [unwired: 2 in]
                                }
                                }
                                n284 = call "headingoperater.vi"("h1"=w502, "h2"=w504) -> ("h2-h1"=w507:dbl)  [unwired: 8 in, 1 out]
                                n285 = call "rotm_siso.vi"("angle[rad]"=w502, "y0"=w500, "x0"=w501, "y"=w505, "x"=w506) -> ("y'"=w512:dbl, "x'"=w499:dbl)  [unwired: 5 in]
                                n286 = call "cubic.vi"("h"=w507, "y"=w512, "x"=w499) -> ("b"=w509:dbl, "a"=w508:dbl)  [unwired: 5 in, 2 out]
                                n287 = Multiply(x=w499, y=0.1) -> (x*y=w498:dbl)
                                n288 = Build Array(w501, w500, w502, w498, w508, w509, 5.0 ("element"), 0.0 ("element")) -> (w503:dbl[])
                                }
                              }
                              n289 = flat-sequence {
                                tunnel: [w530] -> w496
                                frame #0 {
                                n290 = flat-sequence {
                                tunnel: [w546] -> w533
                                tunnel: [w545] -> w532
                                tunnel: [w544] -> w531
                                tunnel: [w543] -> w529
                                tunnel: [w542] -> w528
                                tunnel: [w541] -> w527
                                frame #0 {
                                n291 = disable-structure shown="Enabled" {
                                disable-tunnel: [w554 w559] -> w543
                                disable-tunnel: [w552 w558] -> w542
                                disable-tunnel: [w551 w557] -> w541
                                frame Enabled {
                                n292 = global read "G_NAV.vi" "M6006"() -> (w553:T2)
                                n293 = Unbundle By Name(w553) -> ("lcc[1]"=w552:dbl, "lcc[0]"=w551:dbl, "attitude[2]"=w556:dbl)
                                n294 = call "headingoperater.vi"("h1"=w556, "h2"=1.5707963267948966) -> ("h2-h1"=w554:dbl)  [unwired: 8 in, 1 out]
                                }
                                frame Disabled {
                                n295 = global read "G_VEH.vi" "xyhc"() -> (w560:T3)
                                n296 = Unbundle By Name(w560) -> ("x"=w558:dbl, "y"=w557:dbl, "h"=w559:dbl)
                                }
                                }
                                n297 = local read "parkingpoint"() -> (w548:dbl[][])
                                n298 = Index Array(array=w548, index (row)=4 ("index")) -> (element=w547:dbl[])  [unwired: 1 in]
                                n299 = Index Array(array=w547, index #1=0 ("index")) -> (element #1=w546:dbl, element #2=w545:dbl, element #3=w544:dbl)  [unwired: 2 in]
                                }
                                }
                                n300 = call "headingoperater.vi"("h1"=w529, "h2"=w531) -> ("h2-h1"=w534:dbl)  [unwired: 8 in, 1 out]
                                n301 = call "rotm_siso.vi"("angle[rad]"=w529, "y0"=w527, "x0"=w528, "y"=w532, "x"=w533) -> ("y'"=w540:dbl, "x'"=w539:dbl)  [unwired: 5 in]
                                n302 = call "cubic.vi"("h"=w534, "y"=w540, "x"=w539) -> ("b"=w536:dbl, "a"=w535:dbl)  [unwired: 5 in, 2 out]
                                n303 = Build Array(w528, w527, w529, w539, w535, w536, 5.0 ("element"), 0.0 ("element")) -> (w530:dbl[])
                                }
                              }
                              n304 = Build Array(w496) -> (w495:dbl[][])
                              n305 = Transpose 2D Array(2D array=w495) -> (transposed array=w494:dbl[][])
                              n306 = global write "G_PATH.vi" "path"(w494) -> ()
                              n307 = global write "G_PATH.vi" "path_origin"(w494) -> ()
                            }
                            frame #1 {
                              n308 = call "whereami.vi"() -> ()  [unwired: 12 in]
                            }
                            frame #2 {
                            }
                          }
                          n309 = Array Size(array=w493) -> (size(s)=w492:i32[])
                          n310 = Index Array(array=w485, index (row)=2 ("index")) -> (element=w483:dbl[])  [unwired: 1 in]
                          n311 = global read "G_VEH.vi" "xparking"() -> (w482:T3)
                          n312 = Index Array(array=w483, index #1=0 ("index")) -> (element #1=w480:dbl, element #2=w479:dbl, element #3=w478:dbl)  [unwired: 2 in]
                          n313 = Index Array(array=w492, index=0) -> (element=w490:i32)
                          n314 = Decrement(x=w490) -> (x-1=w489:i32)
                          n315 = for {
                            N: w489 -> [_]
                            tunnel: [w572] -> w488 mode=indexing
                            i -> [w580]
                            w586 = 2 ("disabled index (col)")
                            n316 = local read "parkingpoint"() -> (w588:dbl[][])
                            n317 = Increment(x=w580) -> (x+1=w587:i32)
                            n318 = Index Array(array=w588, index (row) #1=w580, index (row) #2=w587, index (row) #3=w580, index (row) #4=w587, index (col) #4=w586, index (row) #5=w580, index (col) #5=w586) -> (element #1=w579:dbl[], element #2=w570:dbl[], element #3=w566:dbl[], element #4=w585:dbl, element #5=w584:dbl)  [unwired: 3 in]
                            n319 = Index Array(array=w570, index #1=0 ("index")) -> (element #1=w569:dbl, element #2=w568:dbl)  [unwired: 1 in]
                            n320 = Index Array(array=w566, index #1=0 ("index")) -> (element #1=w565:dbl, element #2=w561:dbl, element #3=w562:dbl)  [unwired: 2 in]
                            n321 = call "headingoperater.vi"("h1"=w584, "h2"=w585) -> ("h2-h1"=w583:dbl)  [unwired: 8 in, 1 out]
                            n322 = call "rotm_siso.vi"("angle[rad]"=w562, "y0"=w561, "x0"=w565, "y"=w568, "x"=w569) -> ("y'"=w563:dbl, "x'"=w564:dbl)  [unwired: 5 in]
                            n323 = call "cubic.vi"("h"=w583, "y"=w563, "x"=w564) -> ("b"=w581:dbl, "a"=w582:dbl)  [unwired: 5 in, 2 out]
                            n324 = Index Array(array=w579, index #1=0 ("index")) -> (element #1=w577:dbl, element #2=w576:dbl, element #3=w575:dbl)  [unwired: 2 in]
                            n325 = Build Array(w577, w576, w575, w564, w582, w581, -5.0 ("element"), 0.0 ("element")) -> (w572:dbl[])
                          }
                          n326 = Bundle By Name(cluster=w482, "idx"=1 ("c_idx"), "x"=w480, "y"=w479, "h"=w478) -> (w477:T3)
                          n327 = global write "G_VEH.vi" "xparking"(w477) -> ()
                          n328 = Transpose 2D Array(2D array=w488) -> (transposed array=w487:dbl[][])
                          n329 = global write "G_PATH.vi" "path_rev"(w487) -> ()
                        }
                      }
                    }
                  }
                }
                frame True {
                }
              }
            }
            frame True {
              n330 = flat-sequence {
                tunnel: [w595] -> w589
                frame #0 {
                  n331 = local read "M6006"() -> (w632:T1)
                  n332 = local read "box"() -> (w594:dbl[][])
                  n333 = Unbundle By Name(w632) -> ("lcc[1]"=w628:sgl, "lcc[0]"=w627:sgl, "attitude[2]"=w631:sgl)
                  n334 = Array Subset(array=w594, length (row)=4 ("length")) -> (w593:dbl[][])  [unwired: 3 in]
                  n335 = Negate(x=w631) -> (-x=w630:sgl)
                  n336 = Index Array(array=w593, index (col) #1=0 ("disabled index (col)")) -> (element #1=w634:dbl[], element #2=w633:dbl[])  [unwired: 3 in]
                  n337 = call "rotm_mimo.vi"("angle[rad]"=w630, "reverse"=TRUE, "y0"=w627, "x0"=w628, "y"=w633, "x"=w634) -> ("Y"=w619:dbl[], "X"=w621:dbl[])  [unwired: 2 in, 2 out]
                  n338 = Subtract(x=w621, y=w628) -> (x-y=w625:dbl[])
                  n339 = Subtract(x=w619, y=w627) -> (x-y=w626:dbl[])
                  n340 = Square(x=w625) -> (x^2=w624:dbl[])
                  n341 = Square(x=w626) -> (x^2=w623:dbl[])
                  n342 = Add(x=w624, y=w623) -> (x+y=w622:dbl[])
                  n343 = Array Max & Min(array=w622) -> (min index (indices)=w620:i32)  [unwired: 3 out]
                  n344 = Delete From Array(array=w621, index=w620) -> (deleted portion=w607:dbl, array with subset deleted=w611:dbl[])  [unwired: 1 in]
                  n345 = Delete From Array(array=w619, index=w620) -> (deleted portion=w599:dbl, array with subset deleted=w603:dbl[])  [unwired: 1 in]
                  n346 = Subtract(x=w611, y=w607) -> (x-y=w615:dbl[])
                  n347 = Subtract(x=w603, y=w599) -> (x-y=w614:dbl[])
                  n348 = Square(x=w615) -> (x^2=w616:dbl[])
                  n349 = Square(x=w614) -> (x^2=w617:dbl[])
                  n350 = Add(x=w616, y=w617) -> (x+y=w618:dbl[])
                  n351 = Array Max & Min(array=w618) -> (max index (indices)=w601:i32, min index (indices)=w600:i32)  [unwired: 2 out]
                  n352 = Add(x=w601, y=w600) -> (x+y=w613:i32)
                  n353 = Subtract(x=3, y=w613) -> (x-y=w602:i32)
                  n354 = Index Array(array=w611, index #1=w602, index #2=w601, index #3=w600) -> (element #1=w610:dbl, element #2=w609:dbl, element #3=w608:dbl)
                  n355 = Index Array(array=w603, index #1=w602, index #2=w601, index #3=w600) -> (element #1=w604:dbl, element #2=w605:dbl, element #3=w606:dbl)
                  n356 = Build Array(w607, w610, w609, w608, w607) -> (w598:dbl[])
                  n357 = Build Array(w599, w604, w605, w606, w599) -> (w597:dbl[])
                  n358 = Build Array(w598, w597) -> (w596:dbl[][])
                  n359 = Transpose 2D Array(2D array=w596) -> (transposed array=w595:dbl[][])
                }
              }
              n360 = global write "G_PATH.vi" "parking_count"(0 ("count")) -> ()
              n361 = local read "max cost"() -> (w590:i32)
              n362 = global write "G_PATH.vi" "parking_cost"(w590) -> ()
              n363 = global write "G_PATH.vi" "wpt_park"(w589) -> ()
            }
          }
        }
      }
    }
    frame #5 {
      n364 = Tick Count (ms)() -> (millisecond timer value=w649:u32)
      n365 = local read "tic"() -> (w647:u32)
      n366 = local read "M6006"() -> (w642:T1)
      n367 = Subtract(x=w649, y=w647) -> (x-y=→"time":u32)
      n368 = local read "parkingpoint"() -> (w638:dbl[][])
      n369 = Unbundle By Name(w642) -> ("lcc[1]"=w644:sgl, "lcc[0]"=w645:sgl, "attitude[2]"=w643:sgl)
      n370 = Negate(x=w643) -> (-x=w646:sgl)
      n371 = Index Array(array=w638, index (col) #1=0 ("disabled index (col)")) -> (element #1=w640:dbl[], element #2=w641:dbl[])  [unwired: 3 in]
      n372 = call "rotm_mimo.vi"("angle[rad]"=w646, "y0"=w645, "x0"=w644, "y"=w641, "x"=w640) -> ("Y"=w636:dbl[], "X"=w637:dbl[])  [unwired: 3 in, 2 out]
    }
    frame #6 {
      n373 = flat-sequence {
        tunnel: [w697] -> w653
        tunnel: w651 -> [w678]
        frame #0 {
          n374 = call "Convert to Dynamic Data11"("Array"=w678) -> ("Dynamic Data Type"=w684:dynamicdata)  [unwired: 3 in]
          n375 = local read "sensor_lane"() -> (w680:dbl[][])
          n376 = local read "sensor_obs"() -> (w679:dbl[][])
          n377 = local read "lane"() -> (w688:dbl[][])
          n378 = local read "obs"() -> (w696:dbl[][])
          n379 = local read "box"() -> (w683:dbl[][])
          n380 = Index Array(array=w688, index (col)=0 ("disabled index (col)")) -> (element=w689:dbl[])  [unwired: 1 in]
          n381 = Index Array(array=w680, index (col)=0 ("disabled index (col)")) -> (element=w692:dbl[])  [unwired: 1 in]
          n382 = Index Array(array=w696, index (col)=0 ("disabled index (col)")) -> (element=w695:dbl[])  [unwired: 1 in]
          n383 = Index Array(array=w679, index (col)=0 ("disabled index (col)")) -> (element=w699:dbl[])  [unwired: 1 in]
          n384 = Index Array(array=w683, index (col)=0 ("disabled index (col)")) -> (element=w681:dbl[])  [unwired: 1 in]
          n385 = call "Convert to Dynamic Data6"("Array"=w689) -> ("Dynamic Data Type"=w687:dynamicdata)  [unwired: 3 in]
          n386 = call "Convert to Dynamic Data5"("Array"=w692) -> ("Dynamic Data Type"=w686:dynamicdata)  [unwired: 3 in]
          n387 = call "Convert to Dynamic Data3"("Array"=w695) -> ("Dynamic Data Type"=w694:dynamicdata)  [unwired: 3 in]
          n388 = call "Convert to Dynamic Data"("Array"=w699) -> ("Dynamic Data Type"=w698:dynamicdata)  [unwired: 3 in]
          n389 = call "Convert to Dynamic Data9"("Array"=w681) -> ("Dynamic Data Type"=w685:dynamicdata)  [unwired: 3 in]
          n390 = Merge Signals(w687, w686, w694, w698, w685, w684) -> (w697:dynamicdata)
        }
      }
      n391 = flat-sequence {
        tunnel: [w674] -> w652
        tunnel: w650 -> [w655]
        frame #0 {
          n392 = call "Convert to Dynamic Data12"("Array"=w655) -> ("Dynamic Data Type"=w661:dynamicdata)  [unwired: 3 in]
          n393 = local read "sensor_lane"() -> (w657:dbl[][])
          n394 = local read "sensor_obs"() -> (w656:dbl[][])
          n395 = local read "lane"() -> (w665:dbl[][])
          n396 = local read "obs"() -> (w673:dbl[][])
          n397 = local read "box"() -> (w660:dbl[][])
          n398 = Index Array(array=w665, index (col)=1 ("disabled index (col)")) -> (element=w666:dbl[])  [unwired: 1 in]
          n399 = Index Array(array=w657, index (col)=1 ("disabled index (col)")) -> (element=w669:dbl[])  [unwired: 1 in]
          n400 = Index Array(array=w673, index (col)=1 ("disabled index (col)")) -> (element=w672:dbl[])  [unwired: 1 in]
          n401 = Index Array(array=w656, index (col)=1 ("disabled index (col)")) -> (element=w676:dbl[])  [unwired: 1 in]
          n402 = Index Array(array=w660, index (col)=1 ("disabled index (col)")) -> (element=w658:dbl[])  [unwired: 1 in]
          n403 = call "Convert to Dynamic Data8"("Array"=w666) -> ("Dynamic Data Type"=w664:dynamicdata)  [unwired: 3 in]
          n404 = call "Convert to Dynamic Data7"("Array"=w669) -> ("Dynamic Data Type"=w663:dynamicdata)  [unwired: 3 in]
          n405 = call "Convert to Dynamic Data4"("Array"=w672) -> ("Dynamic Data Type"=w671:dynamicdata)  [unwired: 3 in]
          n406 = call "Convert to Dynamic Data2"("Array"=w676) -> ("Dynamic Data Type"=w675:dynamicdata)  [unwired: 3 in]
          n407 = call "Convert to Dynamic Data10"("Array"=w658) -> ("Dynamic Data Type"=w662:dynamicdata)  [unwired: 3 in]
          n408 = Merge Signals(w664, w663, w671, w675, w662, w661) -> (w674:dynamicdata)
        }
      }
      n409 = call "Build XY Graph"("Y Input"=w652, "X Input"=w653) -> ("XY Graph"=→"XY Graph":cluster{"Y":dbl[], "Y":dbl[]}[])  [unwired: 3 in, 6 out]
    }
  }
